vi "Get Cursor Values from Data.vi"(5 "spectra":cluster{"x0":dbl, "dx":dbl, "Y":dbl[]}[](array[cluster]), 7 "spectra info":T6[](array[typedef]) {"x-axis units" items=["Time (s)"=0, "Frequency-CB (Hz)"=1, "Frequency-CPB (Hz)"=1248, "Frequency-Arbitrary (Hz)"=2357, "Quefrency (s)"=2, "Revolutions (rev)"=3, "Order"=4, "Speed (RPM)"=11, "Speed (rad/s)"=21, "Index"=65535]; "weighting filter" items=["Linear", "A-weighting", "B-weighting", "C-weighting", "ITU-R 468-4", "Dolby", "CCITT", "C-message", "Wb", "Wc", "Wd", "We", "Wf", "Wh", "Wj", "Wk", "Wm", "AES17 20 kHz lowpass", "AES17 40 kHz lowpass", "AES17 20 kHz highpass", "AES17 40 kHz highpass"]; "dB reference [EU]" format="%.2f"; "engineering units" items=["custom..."=0, "V"=1, "A"=21, "C"=30, "pC"=31, "s"=32, "-"=29, "Pa"=2, "N"=20, "g"=3, "m/s^2"=4, "m/s"=5, "m"=6, "mm/s"=12, "mm"=13, "micron/s"=14, "micron"=15, "in/s^2"=7, "in/s"=8, "in"=9, "mil/s"=10, "mil"=11, "rad/s^2"=16, "rad/s"=17, "rad"=18, "deg/s^2"=26, "deg/s"=27, "deg"=28, "RPM"=22, "cycle/s^2"=23, "Hz"=24, "cycle"=25, "strain"=19]; "spectral info"."window" items=["None "=0, "Hanning"=1, "Hamming"=2, "Blackman-Harris"=3, "Exact Blackman"=4, "Blackman"=5, "Flat Top"=6, "4 Term B-Harris "=7, "7 Term B-Harris"=8, "Low Sidelobe"=9, "Force - Exponential"=10, "Gaussian"=62]}, 10 "Refnums for FP Objects":T1, 11 "Display State In":T2={"Graph Visible Items"={"Plot Legend"=FALSE, "Scale Legend"=FALSE, "Graph Palette"=FALSE, "Cursor Legend"=FALSE, "X Scrollbar"=FALSE}, "View Table"=FALSE, "Table Visible Items"={"Vertical Scrollbar"=FALSE, "Horizontal Scrollbar"=FALSE, "Row Headers"=FALSE, "Column Headers"=FALSE, "Vertical Lines"=FALSE, "Horizontal Lines"=FALSE}, "Header Font"={"Font Name"="", "Size"=0, "Bold"=FALSE, "Italic"=FALSE, "Underline"=FALSE, "Strikeout"=FALSE, "Color"=0}, "Cell Font"={"Font Name"="", "Size"=0, "Bold"=FALSE, "Italic"=FALSE, "Underline"=FALSE, "Strikeout"=FALSE, "Color"=0}, "Description and Tip..."={"Description"="", "Tip"=""}, "Moveable Splitter Position"=0, "Measurement Cursor Configuration"={"XY"={"enable XY"=FALSE, "Position (X)"=[], "Type"=enum."Absolute", "Y reference"=0.0, "color"=0}, "band"={"enable band"=FALSE, "B1"=0.0, "B2"=0.0, "Fixed bandwidth (B2-B1)"=0.0, "B1 color"=0, "B2 color"=0}, "harmonic"={"enable harmonics"=FALSE, "X reference (1X)"=0.0, "Maximum"=0, "Subset"=enum."All", "1X color"=0, "MX color"=0}, "sideband"={"enable sideband"=FALSE, "X center (C)"=0.0, "Sidebands"=0, "X spacing (s)"=0.0, "Center color"=0, "Sideband color"=0}}, "Cursors"={"List"=[], "Tags"=[]}, "X Increment"=0.0, "X Scale"={"Label Visible"=FALSE, "Label Text"="", "Mapping Mode"=0, "Format String"=""}, "Y Scale"={"Label Visible"=FALSE, "Label Text"="", "Mapping Mode"=0, "Format String"=""}, "Colors"={"background"=16777215, "major grid"=8355711, "minor grid"=12632256, "font"=0}, "desired spectrum view"={"scaling"={"linear/dB"=enum."no change", "dB reference"=0.0, "power/magnitude"=enum."no change", "view"=enum."no change"}, "spectral density"=enum."no change"}, "Plot Color Wheel"=[3381759, 32768, 982784, 4375295, 13827953, 13457919, 16757522, 4343295, 16728758, 12095254], "Plots"=[], "registered user events"=variant, "Lock 1X to Peak"=FALSE, "spectrum component"=32, "phase spectrum view"={"desired units"=0, "desired wrapping"=4}} caption="State" {"phase spectrum view"."desired wrapping" items=["No change", "Unwrap", "Wrap: -360 to 0", "Wrap: -270 to 90", "Wrap: -180 to 180", "Wrap: -90 to 270", "Wrap: 0 to 360", "Wrap: custom range"]; "phase spectrum view"."desired units" items=["No change", "Radians", "Degrees", "Cycles"]; "spectrum component" items=["Magnitude^2"=37, "Magnitude"=32, "Phase"=33, "Real"=34, "Imaginary"=35, "Coherence"=36, "Unknown"=99]; "Y Scale"."Mapping Mode" items=["Linear", "Logarithmic", "dB"]; "X Scale"."Mapping Mode" items=["Linear", "Logarithmic"]}) -> (2 "value table":string[][](array[string]), 3 "Display State Out":T2={"Graph Visible Items"={"Plot Legend"=FALSE, "Scale Legend"=FALSE, "Graph Palette"=FALSE, "Cursor Legend"=FALSE, "X Scrollbar"=FALSE}, "View Table"=FALSE, "Table Visible Items"={"Vertical Scrollbar"=FALSE, "Horizontal Scrollbar"=FALSE, "Row Headers"=FALSE, "Column Headers"=FALSE, "Vertical Lines"=FALSE, "Horizontal Lines"=FALSE}, "Header Font"={"Font Name"="", "Size"=0, "Bold"=FALSE, "Italic"=FALSE, "Underline"=FALSE, "Strikeout"=FALSE, "Color"=0}, "Cell Font"={"Font Name"="", "Size"=0, "Bold"=FALSE, "Italic"=FALSE, "Underline"=FALSE, "Strikeout"=FALSE, "Color"=0}, "Description and Tip..."={"Description"="", "Tip"=""}, "Moveable Splitter Position"=0, "Measurement Cursor Configuration"={"XY"={"enable XY"=FALSE, "Position (X)"=[], "Type"=enum."Absolute", "Y reference"=0.0, "color"=0}, "band"={"enable band"=FALSE, "B1"=0.0, "B2"=0.0, "Fixed bandwidth (B2-B1)"=0.0, "B1 color"=0, "B2 color"=0}, "harmonic"={"enable harmonics"=FALSE, "X reference (1X)"=0.0, "Maximum"=0, "Subset"=enum."All", "1X color"=0, "MX color"=0}, "sideband"={"enable sideband"=FALSE, "X center (C)"=0.0, "Sidebands"=0, "X spacing (s)"=0.0, "Center color"=0, "Sideband color"=0}}, "Cursors"={"List"=[], "Tags"=[]}, "X Increment"=0.0, "X Scale"={"Label Visible"=FALSE, "Label Text"="", "Mapping Mode"=0, "Format String"=""}, "Y Scale"={"Label Visible"=FALSE, "Label Text"="", "Mapping Mode"=0, "Format String"=""}, "Colors"={"background"=16777215, "major grid"=8355711, "minor grid"=12632256, "font"=0}, "desired spectrum view"={"scaling"={"linear/dB"=enum."no change", "dB reference"=0.0, "power/magnitude"=enum."no change", "view"=enum."no change"}, "spectral density"=enum."no change"}, "Plot Color Wheel"=[3381759, 32768, 982784, 4375295, 13827953, 13457919, 16757522, 4343295, 16728758, 12095254], "Plots"=[], "registered user events"=variant, "Lock 1X to Peak"=FALSE, "spectrum component"=32, "phase spectrum view"={"desired units"=0, "desired wrapping"=4}} caption="State" {"phase spectrum view"."desired wrapping" items=["No change", "Unwrap", "Wrap: -360 to 0", "Wrap: -270 to 90", "Wrap: -180 to 180", "Wrap: -90 to 270", "Wrap: 0 to 360", "Wrap: custom range"]; "phase spectrum view"."desired units" items=["No change", "Radians", "Degrees", "Cycles"]; "spectrum component" items=["Magnitude^2"=37, "Magnitude"=32, "Phase"=33, "Real"=34, "Imaginary"=35, "Coherence"=36, "Unknown"=99]; "Y Scale"."Mapping Mode" items=["Linear", "Logarithmic", "dB"]; "X Scale"."Mapping Mode" items=["Linear", "Logarithmic"]}, 4 "measurement names":string[](array[string]), 6 "channels":string[](array[string]))   [LabVIEW 2017, in "Spectrum with Cursors.xctl"]
doc: "This VI extracts the spectral values at the cursor positions. Based on the spectral data, Row Headers, Column Headers, and Values are written to the table."
uses:
  <vilib>/addons/_XControls/Spectrum with Cursors/Spectrum with Cursors.xctl
  <vilib>/addons/_XControls/Spectrum with Cursors/Controls/State.ctl
  <vilib>/Utility/miscctls.llb/LVFontTypeDef.ctl
  <vilib>/addons/_XControls/Spectrum with Cursors/Controls/Measurement Cursor Configuration.ctl
  <vilib>/addons/_NISVFA/_Shared subVIs/Controls/NI Spectrum Component.ctl
  <vilib>/addons/_NISVFA/_Shared subVIs/Controls/svc_Spectrum Info.ctl
  <vilib>/addons/_NISVFA/_Shared subVIs/Controls/svc_X-Axis Units.ctl
  <vilib>/addons/_NISVFA/_Shared subVIs/Controls/svc_Spectrum Type.ctl
  <vilib>/addons/_NISVFA/_Shared subVIs/Controls/svc_Engineering Units Text Ring.ctl
  <vilib>/addons/_NISVFA/_Shared subVIs/Controls/svc_Weighting Filter Text Ring.ctl
  <vilib>/addons/_NISVFA/_Shared subVIs/Controls/svc_Complimentary Spectrum Units.ctl
  <vilib>/addons/_XControls/Spectrum with Cursors/Controls/Refnums Typedef.ctl
  <vilib>/addons/_NISVFA/_Spectrum Processing/SVFA Get Spectrum Value (N Ch).vi
  <vilib>/Analysis/baseanly.llb/Mean (DBL).vi
  <vilib>/addons/_NISVFA/_Spectrum Processing/SVFA Get Spectrum Subset (N Ch).vi
  <vilib>/addons/_NISVFA/_Spectrum Processing/SVFA Power in Band (N Ch).vi
  <vilib>/addons/_NISVFA/_Spectrum Processing/SVFA Get Spectrum Value (1 Ch).vi
  <vilib>/addons/_NISVFA/_Spectrum Processing/SVFA Get Spectrum Subset (1 Ch).vi
  <vilib>/addons/_NISVFA/_Spectrum Processing/SVFA Power in Band (1 Ch).vi
  <vilib>/addons/_NISVFA/_Spectrum Processing/SVFA Unit Conversion.vi
  <vilib>/addons/_NISVFA/_Spectrum Processing/SVFA Unit Conversion (1 Ch).vi
  <vilib>/addons/_NISVFA/_Spectrum Processing/subVIs/svfa_Conversion Utility (spectrum info).vi
  <vilib>/addons/_NISVFA/_Spectrum Processing/subVIs/svfa_Peak to RMS to Peak2Peak.vi
  <vilib>/addons/_NISVFA/_Spectrum Processing/subVIs/svfa_Mag to Mag2.vi
  <vilib>/addons/_NISVFA/_Spectrum Processing/subVIs/svfa_Linear to dB.vi
  <vilib>/addons/_NISVFA/_Spectrum Processing/subVIs/svfa_dBrefA to dBrefB.vi
  <vilib>/addons/_NISVFA/_Spectrum Processing/subVIs/svfa_Spectrum to Spectral Density.vi
  <vilib>/addons/_NISVFA/_Shared subVIs/Common/svc_Caller VI Returned in Error Source.vi
  <vilib>/addons/_NISVFA/_Shared subVIs/Common/svc_Build Unit Label for Frequency Range.vi
  <vilib>/addons/_NISVFA/_Shared subVIs/Common/svc_Convert Frequency to Frequency String.vi
  <vilib>/addons/_NISVFA/_Shared subVIs/Common/svc_Check Frequency Range in Spectrum.vi
  <vilib>/addons/_NISVFA/_Shared subVIs/Common/svc_Get Weighting Enum and Labels.vi
  <vilib>/addons/_NISVFA/_Shared subVIs/Common/svc_Unit Label Lexical Class.vi
  <vilib>/addons/_NISVFA/_Shared subVIs/Common/svc_Engineering Units to Unit Label.vi
  <vilib>/addons/_NISVFA/_Shared subVIs/Common/svc_Format Value (DBL).vi
  <vilib>/Analysis/NI_AALBase.lvlib
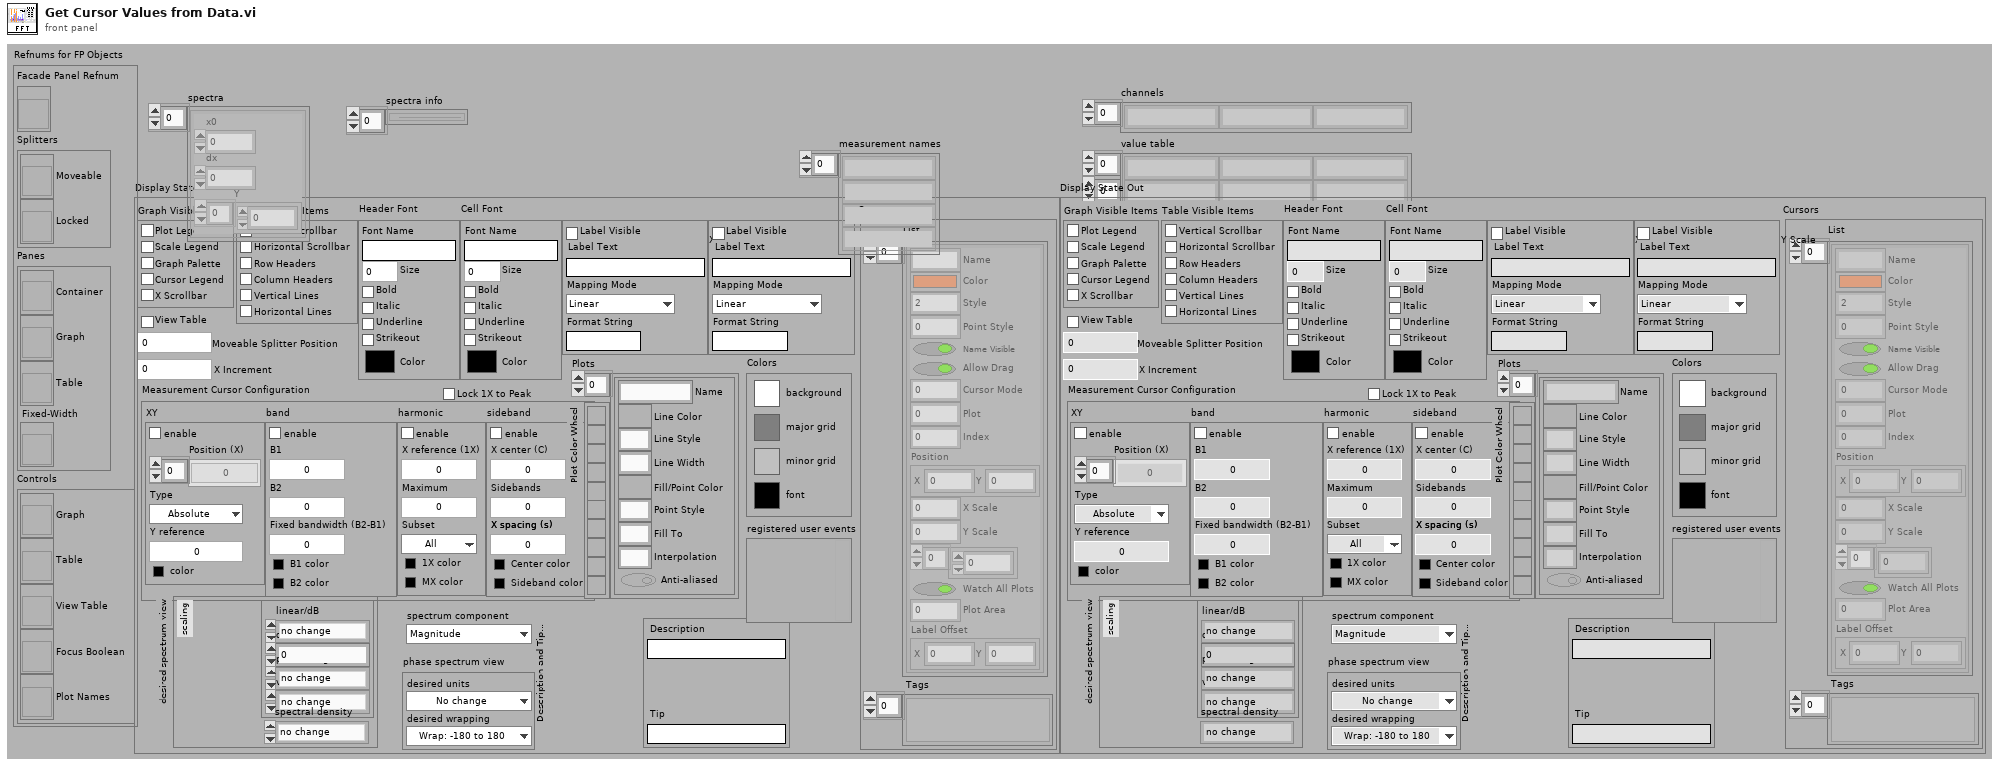
[diagram p1: front panel]
types:
  T1 = typedef "Spectrum with Cursors.xctl/Refnums Typedef.ctl" = cluster{"Facade Panel Refnum":refnum<vi>, "Splitters":cluster{"Moveable":refnum<vi>, "Locked":refnum<vi>}, "Panes":cluster{"Container":refnum<vi>, "Graph":refnum<vi>, "Table":refnum<vi>, "Fixed-Width":refnum<vi>}, "Controls":cluster{"Graph":refnum<vi>, "Table":refnum<vi>, "View Table":refnum<vi>, "Focus Boolean":refnum<vi>, "Plot Names":refnum<vi>}}
  T2 = typedef "Spectrum with Cursors.xctl/State.ctl" = cluster{"Graph Visible Items":cluster{"Plot Legend":bool, "Scale Legend":bool, "Graph Palette":bool, "Cursor Legend":bool, "X Scrollbar":bool}, "View Table":bool, "Table Visible Items":cluster{"Vertical Scrollbar":bool, "Horizontal Scrollbar":bool, "Row Headers":bool, "Column Headers":bool, "Vertical Lines":bool, "Horizontal Lines":bool}, "Header Font":T3, "Cell Font":T3, "Description and Tip...":cluster{"Description":string, "Tip":string}, "Moveable Splitter Position":i32, "Measurement Cursor Configuration":T4, "Cursors":cluster{"List":cluster{"Name":string, "Color":u32, "Style":i32, "Point Style":u8, "Name Visible":bool, "Allow Drag":bool, "Cursor Mode":u32, "Plot":i32, "Index":i32, "Position":cluster{"X":dbl, "Y":dbl}, "X Scale":u32, "Y Scale":u32, "Watch Plots":i32[], "Watch All Plots":bool, "Plot Area":i32, "Label Offset":cluster{"X":dbl, "Y":dbl}}[], "Tags":variant[]}, "X Increment":dbl, "X Scale":cluster{"Label Visible":bool, "Label Text":string, "Mapping Mode":u8, "Format String":string}, "Y Scale":cluster{"Label Visible":bool, "Label Text":string, "Mapping Mode":u8, "Format String":string}, "Colors":cluster{"background":u32, "major grid":u32, "minor grid":u32, "font":u32}, "desired spectrum view":cluster{"scaling":cluster{"linear/dB":enum16{"no change", "linear", "dB"}, "dB reference":dbl, "power/magnitude":enum16{"no change", "power", "magnitude"}, "view":enum16{"no change", "rms", "peak", "peak-peak"}}, "spectral density":enum16{"no change", "spectrum", "spectral density"}}, "Plot Color Wheel":u32[], "Plots":cluster{"Name":string, "Line Color":u32, "Line Style":u8, "Line Width":u8, "Fill/Point Color":u32, "Point Style":u8, "Fill To":i16, "Interpolation":u8, "Anti-aliased":bool}[], "registered user events":variant, "Lock 1X to Peak":bool, "spectrum component":T5, "phase spectrum view":cluster{"desired units":u16, "desired wrapping":u16}}
  T3 = typedef "LVFontTypeDef.ctl" = cluster{"Font Name":string, "Size":u16, "Bold":bool, "Italic":bool, "Underline":bool, "Strikeout":bool, "Color":u32}
  T4 = typedef "Spectrum with Cursors.xctl/Measurement Cursor Configuration.ctl" = cluster{"XY":cluster{"enable XY":bool, "Position (X)":dbl[], "Type":enum16{"Absolute", "Relative"}, "Y reference":dbl, "color":u32}, "band":cluster{"enable band":bool, "B1":dbl, "B2":dbl, "Fixed bandwidth (B2-B1)":dbl, "B1 color":u32, "B2 color":u32}, "harmonic":cluster{"enable harmonics":bool, "X reference (1X)":dbl, "Maximum":i32, "Subset":enum16{"All", "Even", "Odd"}, "1X color":u32, "MX color":u32}, "sideband":cluster{"enable sideband":bool, "X center (C)":dbl, "Sidebands":i32, "X spacing (s)":dbl, "Center color":u32, "Sideband color":u32}}
  T5 = typedef "NI Spectrum Component.ctl" = u16
  T6 = typedef "svc_Spectrum Info.ctl" = cluster{"channel name":string, "description":string, "x-axis units":T7, "spectral info":cluster{"spectrum type":T8, "linear/dB":enum16{"linear", "dB"}, "window":u16, "window size":i32, "FFT size":i32}, "engineering units":T9, "custom label":string, "dB reference [EU]":dbl, "peak units":enum16{"rms", "peak", "peak-peak"}, "weighting filter":T10, "spectral density?":bool, "unit label":string, "spectrum skewed?":bool, "complimentary spectrum units":T11}
  T7 = typedef "svc_X-Axis Units.ctl" = u16
  T8 = typedef "svc_Spectrum Type.ctl" = enum16{"FFT Spectrum [complex]", "Amplitude [Magnitude]", "Power [Magnitude^2]", "Cross Spectrum [complex]", "Frequency Response [Complex]"}
  T9 = typedef "svc_Engineering Units Text Ring.ctl" = u16
  T10 = typedef "svc_Weighting Filter Text Ring.ctl" = u16
  T11 = typedef "svc_Complimentary Spectrum Units.ctl" = enum16{"none", "radians", "degrees", "cycles", "imaginary"}
  T12 = enum16{"coerce to nearest", "coerce to next highest", "coerce to next lowest", "interpolate"}
  T13 = typedef "NI_AALPro.lvlib/windowTd.ctl" = u32
  T14 = cluster{"List":cluster{"Name":string, "Color":u32, "Style":i32, "Point Style":u8, "Name Visible":bool, "Allow Drag":bool, "Cursor Mode":u32, "Plot":i32, "Index":i32, "Position":cluster{"X":dbl, "Y":dbl}, "X Scale":u32, "Y Scale":u32, "Watch Plots":i32[], "Watch All Plots":bool, "Plot Area":i32, "Label Offset":cluster{"X":dbl, "Y":dbl}}[], "Tags":variant[]}
  T15 = cluster{"Name":string, "Color":u32, "Style":i32, "Point Style":u8, "Name Visible":bool, "Allow Drag":bool, "Cursor Mode":u32, "Plot":i32, "Index":i32, "Position":cluster{"X":dbl, "Y":dbl}, "X Scale":u32, "Y Scale":u32, "Watch Plots":i32[], "Watch All Plots":bool, "Plot Area":i32, "Label Offset":cluster{"X":dbl, "Y":dbl}}[]
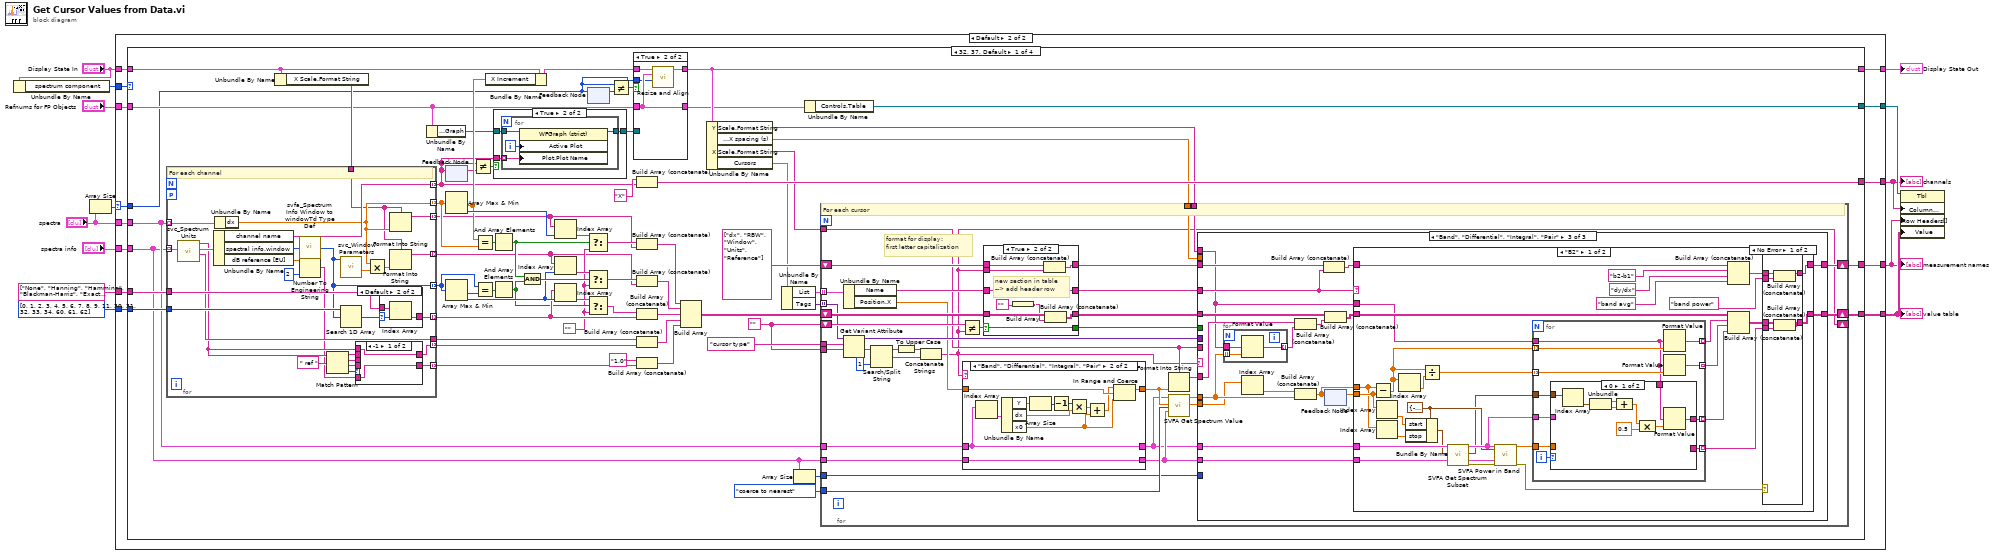
[diagram p0: block diagram]
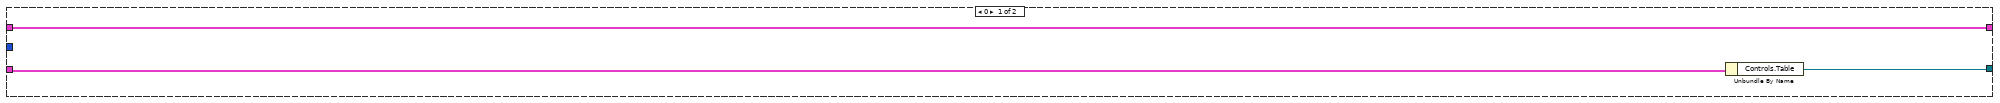
[diagram p2: hidden frame]
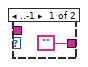
[diagram p6: hidden frame]
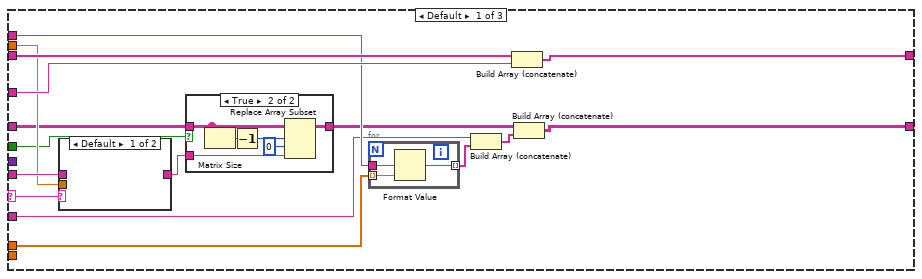
[diagram p9: hidden frame]
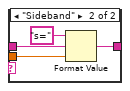
[diagram p11: hidden frame]
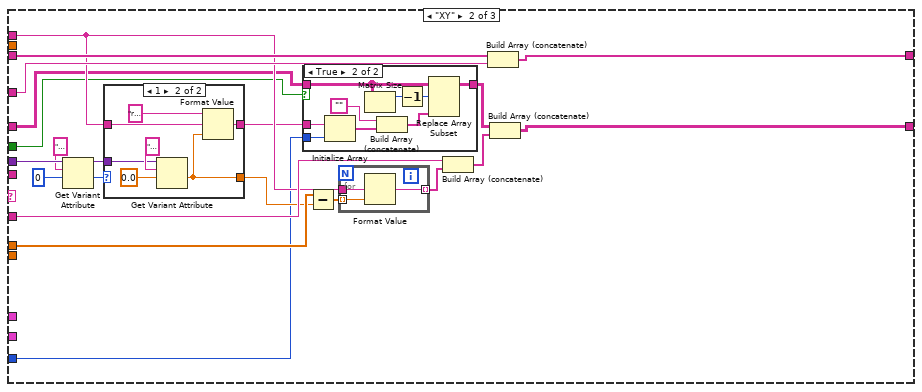
[diagram p12: hidden frame]
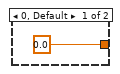
[diagram p14: hidden frame]
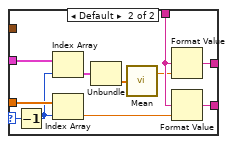
[diagram p16: hidden frame]
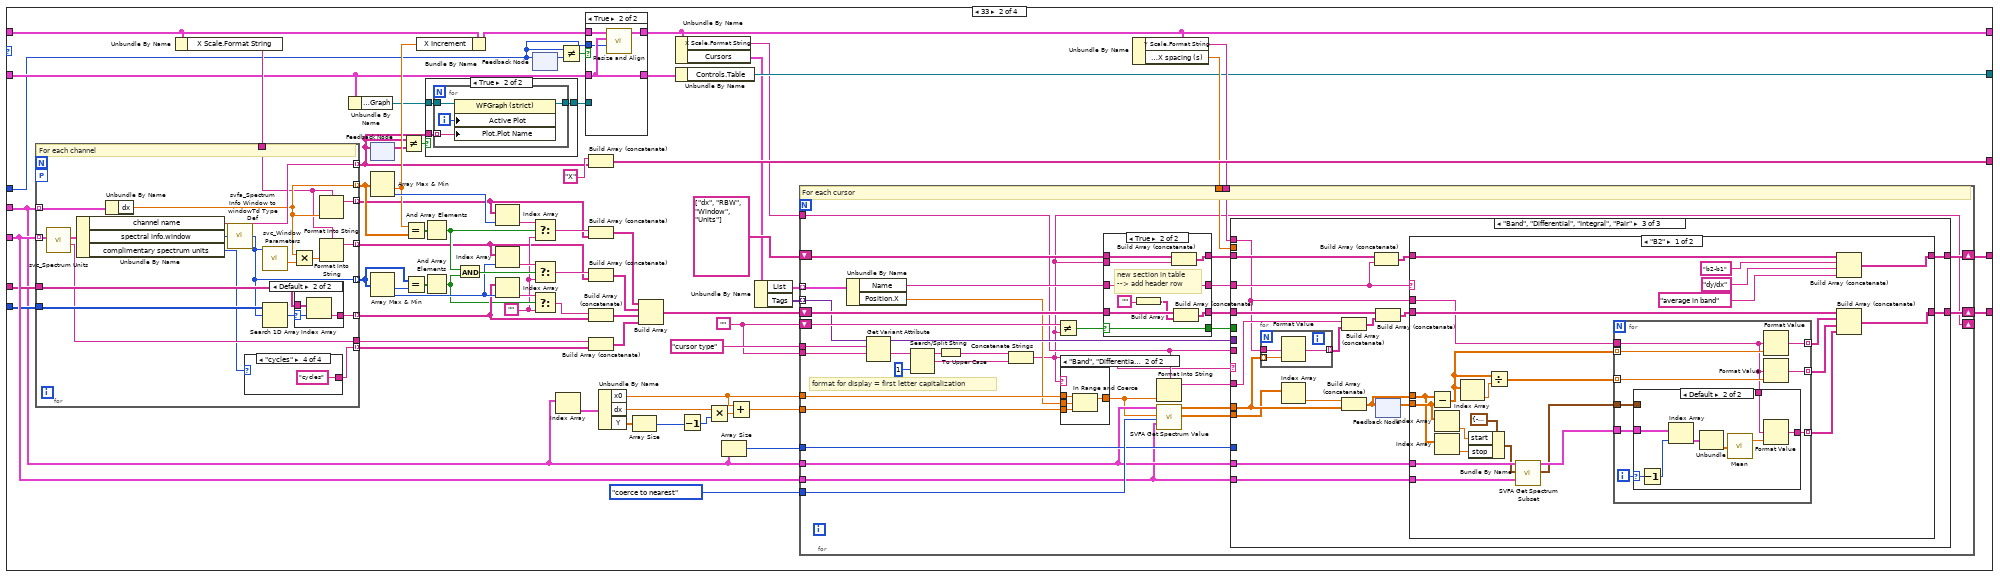
[diagram p18: hidden frame]
diagram:
  n1 = Unbundle By Name("Display State In") -> ("spectrum component"=w2:T5)
  n2 = Array Size(array="spectra") -> (size(s)=w7:i32)
  n3 = case shown="Default" w7 {
    selector: w7 -> [_ w18]
    tunnel: "spectra info" -> [_ w29]
    tunnel: u32[] [0, 1, 2, 3, 4, 5, 6, 7, 8, 9, 11, 30, 31, 32, 33, 34, 60, 61, 62] ("Array") -> [_ w28]
    tunnel: string[] ["None", "Hanning", "Hamming", "Blackman-Harris", "Exact Blackman", "Blackman", "Flat Top", "4 Term B-Harris ", "7 Term B-Harris", "Low Sidelobe", "Blackman Nuttall", "Triangle", "Bartlett-Hanning", "Bohman", "Parzen", "Welch", "Kaiser", "Dolph-Chebyshev", "Gaussian"] ("Array") -> [_ w27]
    tunnel: [_ w26] -> w4
    tunnel: [_ w25] -> w3
    tunnel: [_ w24] -> w5
    tunnel: [w16 w20] -> w10
    tunnel: "spectra" -> [_ w23]
    tunnel: "Display State In" -> [w16 w21]
    tunnel: "Refnums for FP Objects" -> [w15 w19]
    tunnel: [w14 w22] -> w6
    tunnel: w2 -> [_ w17]
    frame 0 {
      n4 = Unbundle By Name(w15) -> ("Controls.Table"=w14:refnum<vi>)
    }
    frame Default {
      n5 = case shown="32, 37, Default" w17 {
        tunnel: w29 -> [w32 w443 w753 w1061]
        tunnel: w28 -> [w93 w442 w752 w1060]
        tunnel: w27 -> [w92 w441 w751 w1059]
        tunnel: [w82 w431 w741 w1049] -> w26
        tunnel: [w81 w430 w740 w1048] -> w25
        tunnel: [w80 w429 w739 w1047] -> w24
        tunnel: w23 -> [w74 w415 w725 w1031]
        tunnel: [w51 w393 w703 w1008] -> w22
        tunnel: w21 -> [w48 w390 w700 w1005]
        tunnel: [w46 w388 w698 w1003] -> w20
        tunnel: w19 -> [w45 w387 w697 w1002]
        tunnel: w18 -> [w41 w383 w693 w998]
        frame 32, 37, Default {
          w79 = "" ("String")
          w56 = "" ("String")
          n6 = Unbundle By Name(w48) -> ("X Scale.Format String"=w50:string)
          n7 = for {
            tunnel: w32 -> [w135] mode=indexing
            tunnel: [w112] -> w33 mode=indexing
            tunnel: w74 -> [w136] mode=indexing
            tunnel: [w116] -> w89 mode=indexing
            tunnel: w93 -> [w132]
            tunnel: w92 -> [w129]
            tunnel: [w128] -> w36 mode=indexing
            tunnel: [w126] -> w37 mode=indexing
            tunnel: [w125] -> w60 mode=indexing
            tunnel: [w124] -> w90
            tunnel: [w114] -> w77 mode=indexing
            tunnel: w50 -> [w110]
            tunnel: [w111] -> w66 mode=indexing
            tunnel: [w109] -> w53 mode=indexing
            workers-P: _ -> [_]
            # "For each channel"
            n8 = call <vilib>:"svc_Spectrum Units.vi"("spectrum info in"=w135) -> ("x-axis unit label"=w124:string, "spectrum info out"=w134:T6, "unit label"=w115:string)  [unwired: 3 in, 1 out]
            n9 = Unbundle By Name(w134) -> ("channel name"=w112:string, "spectral info.window"=w131:u16, "dB reference [EU]"=w122:dbl)
            n10 = Unbundle By Name(w136) -> ("dx"=w111:dbl)
            n11 = call <vilib>:"svfa_Spectrum Info Window to windowTd Type Def.vi"("window"=w131) -> ("window"=w109:T13)  [unwired: 4 in]
            n12 = Number To Engineering String(2:i16 2 ("precision (6)"), 4:w122) -> (0:w113:string)  [unwired: 2 in]
            n13 = Match Pattern(string=w115, regular expression=" ref ") -> (before substring=w119:string, match substring=w118:string, after substring=w117:string, offset past match=w120:i32)  [unwired: 1 in]
            n14 = call <vilib>:"svc_Window Parameters.vi"("window"=w109) -> ("6dB BW"=w133:dbl)  [unwired: 7 in, 3 out]
            n15 = Search 1D Array(1D array=w132, element=w109) -> (index of element=w130:i32)  [unwired: 1 in]
            n16 = case shown="-1" w120 {
              tunnel: w119 -> [_ w140]
              tunnel: w118 -> [_ _]
              tunnel: w117 -> [_ w139]
              tunnel: [w138 w140] -> w116
              tunnel: w115 -> [w138 _]
              tunnel: [w137 w139] -> w114
              tunnel: w113 -> [w137 _]
              frame -1 {
              }
              frame Default {
              }
            }
            n17 = Multiply(x=w111, y=w133) -> (x*y=w127:dbl)
            n18 = case shown="Default" w130 {
              selector: w130 -> [_ w144]
              tunnel: w129 -> [_ w143]
              tunnel: ["" ("String") w142] -> w125
              frame ..-1 {
              }
              frame Default {
                n19 = Index Array(array=w143, index=w144) -> (element=w142:string)
              }
            }
            n20 = Format Into String(format string=w110, w111) -> (resulting string=w128:string)  [unwired: 2 in, 1 out]
            n21 = Format Into String(format string=w110, w127) -> (resulting string=w126:string)  [unwired: 2 in, 1 out]
          }
          n22 = Unbundle By Name(w45) -> ("Controls.Graph"=w52:refnum<vi>)
          n23 = feedback #1() -> (w35:string[])  [unwired: 1 in]
          n24 = feedback-in #1(w33) -> ()
          n25 = Array Max & Min(array=w66) -> (min value=w67:dbl, min index (indices)=w72:i32)  [unwired: 2 out]
          n26 = Array Max & Min(array=w53) -> (min value=w70:T13, min index (indices)=w63:i32)  [unwired: 2 out]
          n27 = Not Equal?(x=w33, y=w35) -> (x != y?=w34:bool)
          n28 = Equal?(x=w67, y=w66) -> (x = y?=w68:bool[])
          n29 = Equal?(x=w53, y=w70) -> (x = y?=w69:bool[])
          n30 = Bundle By Name(cluster=w48, "X Increment"=w67) -> (w47:T2)
          n31 = And Array Elements(Boolean array=w68) -> (logical AND=w57:bool)
          n32 = And Array Elements(Boolean array=w69) -> (logical AND=w59:bool)
          n33 = case shown="True" w34 {
            tunnel: w52 -> [w95 w98]
            tunnel: [w95 w97] -> w42
            tunnel: w33 -> [_ w96]
            frame False {
            }
            frame True {
              n34 = for {
                tunnel: w98 -> [w102]
                tunnel: w96 -> [w100] mode=indexing
                tunnel: [w99] -> w97
                i -> [w101]
                n35 = property class="WFGraph (strict)"(reference=w102, "Active Plot"=w101, "Plot.Plot Name"=w100) -> (reference out=w99:refnum<vi>)  [unwired: 1 in, 1 out]
              }
            }
          }
          n36 = And(x=w57, y=w59) -> (x .and. y?=w64:bool)
          n37 = Index Array(array=w36, index=w72) -> (element=w55:string)
          n38 = Index Array(array=w37, index=w63) -> (element=w65:string)
          n39 = Index Array(array=w60, index=w63) -> (element=w61:string)
          n40 = feedback #2() -> (w73:i32)  [unwired: 1 in]
          n41 = feedback-in #2(w41) -> ()
          n42 = Select(t=w55, s=w57, f=w56) -> (s? t:f=w54:string)
          n43 = Select(t=w65, s=w64, f=w56) -> (s? t:f=w62:string)
          n44 = Select(t=w61, s=w59, f=w56) -> (s? t:f=w58:string)
          n45 = Not Equal?(x=w41, y=w73) -> (x != y?=w43:bool)
          n46 = case shown="True" w43 {
            tunnel: w47 -> [w104 w108]
            tunnel: [w104 w107] -> w46
            tunnel: w45 -> [w103 w106]
            tunnel: [w103 w106] -> w44
            tunnel: w41 -> [_ w105]
            tunnel: w42 -> [_ _]
            frame False {
            }
            frame True {
              n47 = call <vilib>:"Resize and Align.vi"("number of channels"=w105, "Refnums for Resizing and Alignment"=w106, "State in"=w108) -> ("State out"=w107:T2)  [unwired: 7 in, 1 out]
            }
          }
          n48 = Build Array (concatenate)("X" ("String"), w33) -> (w80:string[])
          n49 = Build Array (concatenate)(w54, w36) -> (w84:string[])
          n50 = Build Array (concatenate)(w62, w37) -> (w87:string[])
          n51 = Build Array (concatenate)(w58, w60) -> (w83:string[])
          n52 = Build Array (concatenate)(w90, w89) -> (w88:string[])
          n53 = Build Array (concatenate)("1.0" ("String"), w77) -> (w78:string[])
          n54 = Build Array(w84, w87, w83, w88, w78) -> (w76:string[][])
          n55 = Unbundle By Name(w46) -> ("Y Scale.Format String"=w31:string, "Measurement Cursor Configuration.sideband.X spacing (s)"=w30:dbl, "X Scale.Format String"=w49:string, "Cursors"=w40:T14)
          n56 = Unbundle By Name(w40) -> ("List"=w39:T15, "Tags"=w38:variant[])
          n57 = Array Size(array=w32) -> (size(s)=w75:i32)
          n58 = Unbundle By Name(w44) -> ("Controls.Table"=w51:refnum<vi>)
          n59 = for {
            tunnel: w74 -> [w145]
            tunnel: w32 -> [w147]
            tunnel: T12."coerce to nearest" ("frequency coercion") -> [w180]
            shift-right: [w178] -> w81
            shift-left: string[] ["dx", "RBW", "Window", "Units", "Reference"] ("Array") -> [w170]
            shift-right: [w177] -> w82
            shift-left: w76 -> [w171]
            tunnel: "cursor type" -> [w176]
            shift-right: [w149] -> _
            shift-left: w79 -> [w175]
            tunnel: w79 -> [w174]
            tunnel: w49 -> [w150]
            tunnel: w31 -> [w160]
            tunnel: w75 -> [w158]
            tunnel: w30 -> [w157]
            tunnel: w39 -> [w154] mode=indexing
            tunnel: w38 -> [w151] mode=indexing
            # "format for display:\nfirst letter capitalization"
            # "For each cursor"
            n60 = Get Variant Attribute(Variant=w151, name=w176, default value (empty Variant)=w174) -> (duplicate Variant=w162:variant, value=w163:string)  [unwired: 1 in, 2 out]
            n61 = Unbundle By Name(w154) -> ("Name"=w153:string, "Position.X"=w152:dbl)
            n62 = Search/Split String(string=w163, offset (0)=1) -> (substring before match=w166:string, match + rest of string=w164:string)  [unwired: 1 in, 1 out]
            n63 = To Upper Case(1:w166) -> (0:w165:string)
            n64 = Concatenate Strings(w165, w164) -> (w149:string)
            n65 = Not Equal?(x=w175, y=w149) -> (x != y?=w173:bool)
            n66 = case shown="\"Band\", \"Differential\", \"Integral\", \"Pair\"" w149 {
              tunnel: w152 -> [w183 w195]
              tunnel: [w183 w194] -> w155
              tunnel: [w181 w193] -> w148
              tunnel: w147 -> [w181 w193]
              tunnel: [w182 w187] -> w146
              tunnel: w145 -> [w182 w187]
              frame Default {
              }
              frame "Band", "Differential", "Integral", "Pair" {
                n67 = Index Array(array=w187) -> (element=w188:cluster{"x0":dbl, "dx":dbl, "Y":dbl[]})  [unwired: 1 in]
                n68 = Unbundle By Name(w188) -> ("Y"=w189:dbl[], "dx"=w185:dbl, "x0"=w184:dbl)
                n69 = Array Size(array=w189) -> (size(s)=w190:i32)
                n70 = Decrement(x=w190) -> (x-1=w191:i32)
                n71 = Multiply(x=w191, y=w185) -> (x*y=w192:dbl)
                n72 = Add(x=w192, y=w184) -> (x+y=w186:dbl)
                n73 = In Range and Coerce(upper limit=w186, x=w195, lower limit=w184) -> (coerced(x)=w194:dbl)  [unwired: 1 out]
              }
            }
            n74 = case shown="True" w173 {
              selector: w173 -> [w196 w200]
              tunnel: [w199 w208] -> w172
              tunnel: w153 -> [w199 w208]
              tunnel: w171 -> [w197 w203]
              tunnel: w170 -> [w198 w206]
              tunnel: [w198 w207] -> w169
              tunnel: [w197 w204] -> w168
              tunnel: w149 -> [_ w205]
              tunnel: [w196 w200] -> w159
              frame False {
              }
              frame True {
                # "new section in table\n--> add header row"
                n75 = Build Array("") -> (w201:string[])
                n76 = Build Array (concatenate)(w206, w205) -> (w207:string[])
                n77 = Build Array (concatenate)(w203, w201) -> (w204:string[][])
              }
            }
            n78 = Format Into String(format string=w150, w155) -> (resulting string=w161:string)  [unwired: 2 in, 1 out]
            n79 = call-poly <vilib>:"SVFA Get Spectrum Value.vi"("spectra"=w146, "x value (1000)"=w155, "coercion (nearest)"=w180, "spectrum info"=w148) -> ("spectra values"=w179:dbl[], "actual x values"=w156:dbl[])  [unwired: 11 in, 3 out]
            n80 = case shown="\"Band\", \"Differential\", \"Integral\", \"Pair\"" w149 {
              selector: w149 -> [w216 _ _]
              tunnel: w179 -> [w218 w255 w293]
              tunnel: w169 -> [w224 w259 w298]
              tunnel: w172 -> [w223 w258 w292]
              tunnel: [w222 w257 w291] -> w178
              tunnel: w168 -> [w212 w242 w297]
              tunnel: [w221 w256 w288] -> w177
              tunnel: w162 -> [_ w254 _]
              tunnel: w161 -> [w215 w249 w295]
              tunnel: w160 -> [w219 w244 w283]
              tunnel: w159 -> [w210 w243 _]
              tunnel: w158 -> [_ w239 _]
              tunnel: w150 -> [w214 _ _]
              tunnel: w157 -> [w213 _ _]
              tunnel: w156 -> [_ _ w287]
              tunnel: w146 -> [_ _ w282]
              tunnel: w148 -> [_ _ w281]
              frame Default {
                n81 = case shown="Default" w216 {
                  tunnel: w214 -> [_ w234]
                  tunnel: w213 -> [_ w233]
                  tunnel: [_ w232] -> w209
                  frame Default {
                  }
                  frame "Sideband" {
                    n82 = Format Value(string ("")="s=", format string=w234, value (0)=w233) -> (output string=w232:string)
                  }
                }
                n83 = case shown="True" w210 {
                  tunnel: w212 -> [w225 w229]
                  tunnel: [w225 w231] -> w211
                  tunnel: w209 -> [_ w227]
                  frame False {
                  }
                  frame True {
                    n84 = Matrix Size(0:w229) -> (1:w230:i32)  [unwired: 1 out]
                    n85 = Decrement(x=w230) -> (x-1=w228:i32)
                    n86 = Replace Array Subset(array=w229, new element=w227, index (row)=w228, index (col)=0 ("disabled index (col)")) -> (w231:string[][])
                  }
                }
                n87 = for {
                  tunnel: w218 -> [w238] mode=indexing
                  tunnel: [w237] -> w220 mode=indexing
                  tunnel: w219 -> [w236]
                  n88 = Format Value(format string=w236, value (0)=w238) -> (output string=w237:string)  [unwired: 1 in]
                }
                n89 = Build Array (concatenate)(w215, w220) -> (w217:string[])
                n90 = Build Array (concatenate)(w224, w223) -> (w222:string[])
                n91 = Build Array (concatenate)(w211, w217) -> (w221:string[][])
              }
              frame "XY" {
                n92 = Get Variant Attribute(Variant=w254, name="xy type", default value (empty Variant)=u16 0 ("precision (6)")) -> (duplicate Variant=w253:variant, value=w250:u16)  [unwired: 1 in, 2 out]
                n93 = case shown="1" w250 {
                  tunnel: [0.0 ("element") w275] -> w247
                  tunnel: w253 -> [_ w278]
                  tunnel: w244 -> [_ w276]
                  tunnel: [_ w274] -> w240
                  frame 0, Default {
                  }
                  frame 1 {
                    n94 = Get Variant Attribute(Variant=w278, name="y reference", default value (empty Variant)=0.0 ("element")) -> (value=w275:dbl)  [unwired: 1 in, 3 out]
                    n95 = Format Value(string ("")="ref=", format string=w276, value (0)=w275) -> (output string=w274:string)
                  }
                }
                n96 = case shown="True" w243 {
                  tunnel: w242 -> [w260 w265]
                  tunnel: [w260 w269] -> w241
                  tunnel: w240 -> [_ w268]
                  tunnel: w239 -> [_ w267]
                  frame False {
                  }
                  frame True {
                    n97 = Initialize Array(w268, w267) -> (w263:string[])
                    n98 = Matrix Size(0:w265) -> (1:w266:i32)  [unwired: 1 out]
                    n99 = Build Array (concatenate)("", w263) -> (w261:string[])
                    n100 = Decrement(x=w266) -> (x-1=w264:i32)
                    n101 = Replace Array Subset(array=w265, new element=w261, index (row)=w264) -> (w269:string[][])  [unwired: 1 in]
                  }
                }
                n102 = Subtract(x=w255, y=w247) -> (x-y=w246:dbl[])
                n103 = for {
                  tunnel: w246 -> [w272] mode=indexing
                  tunnel: [w271] -> w245 mode=indexing
                  tunnel: w244 -> [w270]
                  n104 = Format Value(format string=w270, value (0)=w272) -> (output string=w271:string)  [unwired: 1 in]
                }
                n105 = Build Array (concatenate)(w249, w245) -> (w248:string[])
                n106 = Build Array (concatenate)(w259, w258) -> (w257:string[])
                n107 = Build Array (concatenate)(w241, w248) -> (w256:string[][])
              }
              frame "Band", "Differential", "Integral", "Pair" {
                n108 = for {
                  tunnel: w293 -> [w374] mode=indexing
                  tunnel: [w373] -> w296 mode=indexing
                  tunnel: w283 -> [w372]
                  n109 = Format Value(format string=w372, value (0)=w374) -> (output string=w373:string)  [unwired: 1 in]
                }
                n110 = Index Array(array=w287) -> (element=w286:dbl)  [unwired: 1 in]
                n111 = Build Array (concatenate)(w295, w296) -> (w294:string[])
                n112 = Build Array (concatenate)(w286, w293) -> (w285:dbl[])
                n113 = Build Array (concatenate)(w298, w292) -> (w290:string[])
                n114 = Build Array (concatenate)(w297, w294) -> (w289:string[][])
                n115 = feedback-in #3(w285) -> ()
                n116 = feedback #3() -> (w284:dbl[])  [unwired: 1 in]
                n117 = case shown="\"B2\"" w292 {
                  tunnel: [w305 w371] -> w291
                  tunnel: w290 -> [w330 w371]
                  tunnel: w289 -> [w328 w370]
                  tunnel: [w302 w370] -> w288
                  tunnel: w285 -> [w314 _]
                  tunnel: w284 -> [w316 _]
                  tunnel: w283 -> [w326 _]
                  tunnel: w282 -> [w320 _]
                  tunnel: w281 -> [w319 _]
                  frame "B2" {
                    w309 = cluster{"start":dbl, "stop":dbl} {"start"=-1.0, "stop"=-1.0} ("range")
                    n118 = Subtract(x=w314, y=w316) -> (x-y=w324:dbl[])
                    n119 = Index Array(array=w316) -> (element=w315:dbl)  [unwired: 1 in]
                    n120 = Index Array(array=w314) -> (element=w313:dbl)  [unwired: 1 in]
                    n121 = Index Array(array=w324) -> (element=w325:dbl)  [unwired: 1 in]
                    n122 = Bundle By Name(cluster=w309, "start"=w315, "stop"=w313) -> (w317:cluster{"start":dbl, "stop":dbl})
                    n123 = Divide(x=w324, y=w325) -> (x/y=w323:dbl[])
                    n124 = call-poly <vilib>:"SVFA Get Spectrum Subset.vi"("spectra"=w320, "range"=w317, "spectrum info"=w319) -> ("spectra subsets"=w312:cluster{"x0":dbl, "dx":dbl, "magnitude":dbl[]}[], "actual ranges"=w308:cluster{"start":dbl, "stop":dbl}[], "dup spectrum info"=w318:T6[], "error out"=w299:errorcluster)  [unwired: 11 in, 2 out]
                    n125 = call-poly <vilib>:"SVFA Power in Band.vi"("spectra"=w312, "range"=w309, "spectrum info"=w318, "error in (no error)"=w299) -> ("powers in band"=w311:dbl[], "error out"=w300:errorcluster)  [unwired: 13 in, 1 out]
                    n126 = for {
                      tunnel: w324 -> [w349] mode=indexing
                      tunnel: [w348] -> w327 mode=indexing
                      tunnel: w326 -> [w342]
                      tunnel: w323 -> [w347] mode=indexing
                      tunnel: [w346] -> w322 mode=indexing
                      tunnel: w312 -> [w344]
                      tunnel: w311 -> [w343]
                      tunnel: [w341] -> w301 mode=indexing
                      tunnel: [w340] -> w310 mode=indexing
                      tunnel: w308 -> [w339]
                      i -> [w345]
                      n127 = case shown="0" w345 {
                        selector: w345 -> [_ w369]
                        tunnel: w344 -> [_ w368]
                        tunnel: w343 -> [_ w367]
                        tunnel: w342 -> [w352 w366]
                        tunnel: [_ w364] -> w341
                        tunnel: [w351 w363] -> w340
                        tunnel: w339 -> [w358 _]
                        frame 0 {
                          n128 = Index Array(array=w358) -> (element=w350:cluster{"start":dbl, "stop":dbl})  [unwired: 1 in]
                          n129 = Unbundle(w350) -> ("start"=w357:dbl, "stop"=w356:dbl)
                          n130 = Compound Arithmetic op=ADD(w357, w356) -> (w355:dbl)
                          n131 = Compound Arithmetic op=MULTIPLY(w355, 0.5 ("value")) -> (w353:dbl)
                          n132 = Format Value(format string=w352, value (0)=w353) -> (output string=w351:string)  [unwired: 1 in]
                        }
                        frame Default {
                          n133 = Decrement(x=w369) -> (x-1=w359:i32)
                          n134 = Index Array(array=w368, index=w359) -> (element=w362:cluster{"x0":dbl, "dx":dbl, "magnitude":dbl[]})
                          n135 = Index Array(array=w367, index=w359) -> (element=w365:dbl)
                          n136 = Unbundle(w362) -> ("magnitude"=w361:dbl[])  [unwired: 2 out]
                          n137 = call-poly <vilib>:"Mean.vi"("X"=w361) -> ("mean"=w360:dbl)  [unwired: 1 out]
                          n138 = Format Value(format string=w366, value (0)=w360) -> (output string=w363:string)  [unwired: 1 in]
                          n139 = Format Value(format string=w366, value (0)=w365) -> (output string=w364:string)  [unwired: 1 in]
                        }
                      }
                      n140 = Format Value(format string=w342, value (0)=w349) -> (output string=w348:string)  [unwired: 1 in]
                      n141 = Format Value(format string=w342, value (0)=w347) -> (output string=w346:string)  [unwired: 1 in]
                    }
                    n142 = Build Array (concatenate)(w330, "b2-b1", "dy/dx", "band avg") -> (w306:string[])
                    n143 = Build Array (concatenate)(w328, w327, w322, w310) -> (w303:string[][])
                    n144 = case shown="No Error" w300 {
                      tunnel: w306 -> [w336 w338]
                      tunnel: [w335 w338] -> w305
                      tunnel: "band power" -> [w334 _]
                      tunnel: w303 -> [w333 w337]
                      tunnel: [w332 w337] -> w302
                      tunnel: w301 -> [w331 _]
                      frame No Error {
                        n145 = Build Array (concatenate)(w336, w334) -> (w335:string[])
                        n146 = Build Array (concatenate)(w333, w331) -> (w332:string[][])
                      }
                      frame Error {
                      }
                    }
                  }
                  frame "B1", Default {
                  }
                }
              }
            }
          }
        }
        frame 33 {
          w428 = "" ("String")
          w398 = "" ("String")
          n147 = Unbundle By Name(w390) -> ("X Scale.Format String"=w392:string)
          n148 = for {
            tunnel: w443 -> [w476] mode=indexing
            tunnel: [w464] -> w375 mode=indexing
            tunnel: w415 -> [w477] mode=indexing
            tunnel: [w459] -> w438 mode=indexing
            tunnel: w442 -> [w473]
            tunnel: w441 -> [w470]
            tunnel: [w469] -> w378 mode=indexing
            tunnel: [w467] -> w379 mode=indexing
            tunnel: [w466] -> w402 mode=indexing
            tunnel: [w465] -> w439
            tunnel: w392 -> [w462]
            tunnel: [w463] -> w408 mode=indexing
            tunnel: [w461] -> w395 mode=indexing
            workers-P: _ -> [_]
            # "For each channel"
            n149 = call <vilib>:"svc_Spectrum Units.vi"("spectrum info in"=w476) -> ("x-axis unit label"=w465:string, "spectrum info out"=w475:T6)  [unwired: 3 in, 2 out]
            n150 = Unbundle By Name(w475) -> ("channel name"=w464:string, "spectral info.window"=w472:u16, "complimentary spectrum units"=w460:T11)
            n151 = Unbundle By Name(w477) -> ("dx"=w463:dbl)
            n152 = call <vilib>:"svfa_Spectrum Info Window to windowTd Type Def.vi"("window"=w472) -> ("window"=w461:T13)  [unwired: 4 in]
            n153 = case shown="\"cycles\"" w460 {
              tunnel: ["" ("String") "rad" ("String") "deg" ("String") "cycles" ("String")] -> w459
              frame Default {
              }
              frame "radians" {
              }
              frame "degrees" {
              }
              frame "cycles" {
              }
            }
            n154 = call <vilib>:"svc_Window Parameters.vi"("window"=w461) -> ("6dB BW"=w474:dbl)  [unwired: 7 in, 3 out]
            n155 = Search 1D Array(1D array=w473, element=w461) -> (index of element=w471:i32)  [unwired: 1 in]
            n156 = Multiply(x=w463, y=w474) -> (x*y=w468:dbl)
            n157 = case shown="Default" w471 {
              selector: w471 -> [_ w485]
              tunnel: w470 -> [_ w484]
              tunnel: ["" ("String") w483] -> w466
              frame ..-1 {
              }
              frame Default {
                n158 = Index Array(array=w484, index=w485) -> (element=w483:string)
              }
            }
            n159 = Format Into String(format string=w462, w463) -> (resulting string=w469:string)  [unwired: 2 in, 1 out]
            n160 = Format Into String(format string=w462, w468) -> (resulting string=w467:string)  [unwired: 2 in, 1 out]
          }
          n161 = Unbundle By Name(w387) -> ("Controls.Graph"=w394:refnum<vi>)
          n162 = feedback #4() -> (w377:string[])  [unwired: 1 in]
          n163 = feedback-in #4(w375) -> ()
          n164 = Array Max & Min(array=w408) -> (min value=w409:dbl, min index (indices)=w413:i32)  [unwired: 2 out]
          n165 = Array Max & Min(array=w395) -> (min value=w412:T13, min index (indices)=w405:i32)  [unwired: 2 out]
          n166 = Not Equal?(x=w375, y=w377) -> (x != y?=w376:bool)
          n167 = Equal?(x=w409, y=w408) -> (x = y?=w410:bool[])
          n168 = Equal?(x=w395, y=w412) -> (x = y?=w411:bool[])
          n169 = Bundle By Name(cluster=w390, "X Increment"=w409) -> (w389:T2)
          n170 = And Array Elements(Boolean array=w410) -> (logical AND=w399:bool)
          n171 = And Array Elements(Boolean array=w411) -> (logical AND=w401:bool)
          n172 = case shown="True" w376 {
            tunnel: w394 -> [w445 w448]
            tunnel: [w445 w447] -> w384
            tunnel: w375 -> [_ w446]
            frame False {
            }
            frame True {
              n173 = for {
                tunnel: w448 -> [w452]
                tunnel: w446 -> [w450] mode=indexing
                tunnel: [w449] -> w447
                i -> [w451]
                n174 = property class="WFGraph (strict)"(reference=w452, "Active Plot"=w451, "Plot.Plot Name"=w450) -> (reference out=w449:refnum<vi>)  [unwired: 1 in, 1 out]
              }
            }
          }
          n175 = And(x=w399, y=w401) -> (x .and. y?=w406:bool)
          n176 = Index Array(array=w378, index=w413) -> (element=w397:string)
          n177 = Index Array(array=w379, index=w405) -> (element=w407:string)
          n178 = Index Array(array=w402, index=w405) -> (element=w403:string)
          n179 = feedback #5() -> (w414:i32)  [unwired: 1 in]
          n180 = feedback-in #5(w383) -> ()
          n181 = Select(t=w397, s=w399, f=w398) -> (s? t:f=w396:string)
          n182 = Select(t=w407, s=w406, f=w398) -> (s? t:f=w404:string)
          n183 = Select(t=w403, s=w401, f=w398) -> (s? t:f=w400:string)
          n184 = Index Array(array=w415) -> (element=w423:cluster{"x0":dbl, "dx":dbl, "Y":dbl[]})  [unwired: 1 in]
          n185 = Not Equal?(x=w383, y=w414) -> (x != y?=w385:bool)
          n186 = case shown="True" w385 {
            tunnel: w389 -> [w454 w458]
            tunnel: [w454 w457] -> w388
            tunnel: w387 -> [w453 w456]
            tunnel: [w453 w456] -> w386
            tunnel: w383 -> [_ w455]
            tunnel: w384 -> [_ _]
            frame False {
            }
            frame True {
              n187 = call <vilib>:"Resize and Align.vi"("number of channels"=w455, "Refnums for Resizing and Alignment"=w456, "State in"=w458) -> ("State out"=w457:T2)  [unwired: 7 in, 1 out]
            }
          }
          n188 = Build Array (concatenate)("X" ("String"), w375) -> (w429:string[])
          n189 = Build Array (concatenate)(w396, w378) -> (w433:string[])
          n190 = Build Array (concatenate)(w404, w379) -> (w436:string[])
          n191 = Build Array (concatenate)(w400, w402) -> (w432:string[])
          n192 = Build Array (concatenate)(w439, w438) -> (w437:string[])
          n193 = Unbundle By Name(w423) -> ("x0"=w416:dbl, "dx"=w419:dbl, "Y"=w422:dbl[])
          n194 = Array Size(array=w422) -> (size(s)=w421:i32)
          n195 = Build Array(w433, w436, w432, w437) -> (w426:string[][])
          n196 = Unbundle By Name(w388) -> ("X Scale.Format String"=w391:string, "Cursors"=w382:T14)
          n197 = Unbundle By Name(w386) -> ("Controls.Table"=w393:refnum<vi>)
          n198 = Decrement(x=w421) -> (x-1=w420:i32)
          n199 = Multiply(x=w419, y=w420) -> (x*y=w418:dbl)
          n200 = Array Size(array=w415) -> (size(s)=w425:i32)
          n201 = Add(x=w416, y=w418) -> (x+y=w417:dbl)
          n202 = Unbundle By Name(w382) -> ("List"=w381:T15, "Tags"=w380:variant[])
          n203 = Unbundle By Name(w388) -> ("Y Scale.Format String"=w427:string, "Measurement Cursor Configuration.sideband.X spacing (s)"=w424:dbl)
          n204 = for {
            tunnel: w415 -> [w496]
            tunnel: w443 -> [w495]
            tunnel: T12."coerce to nearest" ("frequency coercion") -> [w521]
            shift-right: [w519] -> w430
            shift-left: string[] ["dx", "RBW", "Window", "Units"] ("Array") -> [w511]
            shift-right: [w518] -> w431
            shift-left: w426 -> [w512]
            tunnel: "cursor type" -> [w517]
            shift-right: [w486] -> _
            shift-left: w428 -> [w516]
            tunnel: w428 -> [w515]
            tunnel: w391 -> [w487]
            tunnel: w427 -> [w501]
            tunnel: w425 -> [w499]
            tunnel: w424 -> [w498]
            tunnel: w417 -> [w493]
            tunnel: w416 -> [w492]
            tunnel: w381 -> [w491] mode=indexing
            tunnel: w380 -> [w488] mode=indexing
            # "format for display = first letter capitalization"
            # "For each cursor"
            n205 = Unbundle By Name(w491) -> ("Name"=w490:string, "Position.X"=w489:dbl)
            n206 = Get Variant Attribute(Variant=w488, name=w517, default value (empty Variant)=w515) -> (duplicate Variant=w503:variant, value=w504:string)  [unwired: 1 in, 2 out]
            n207 = Search/Split String(string=w504, offset (0)=1) -> (substring before match=w507:string, match + rest of string=w505:string)  [unwired: 1 in, 1 out]
            n208 = To Upper Case(1:w507) -> (0:w506:string)
            n209 = Concatenate Strings(w506, w505) -> (w486:string)
            n210 = Not Equal?(x=w516, y=w486) -> (x != y?=w514:bool)
            n211 = case shown="\"Band\", \"Differential\", \"Integral\", \"Pair\"" w486 {
              tunnel: w489 -> [w522 w526]
              tunnel: [w522 w525] -> w494
              tunnel: w493 -> [_ w524]
              tunnel: w492 -> [_ w523]
              frame Default {
              }
              frame "Band", "Differential", "Integral", "Pair" {
                n212 = In Range and Coerce(upper limit=w523, x=w526, lower limit=w524) -> (coerced(x)=w525:dbl)  [unwired: 1 out]
              }
            }
            n213 = case shown="True" w514 {
              selector: w514 -> [w527 w531]
              tunnel: [w530 w539] -> w513
              tunnel: w490 -> [w530 w539]
              tunnel: w512 -> [w528 w534]
              tunnel: w511 -> [w529 w537]
              tunnel: [w529 w538] -> w510
              tunnel: [w528 w535] -> w509
              tunnel: w486 -> [_ w536]
              tunnel: [w527 w531] -> w500
              frame False {
              }
              frame True {
                # "new section in table\n--> add header row"
                n214 = Build Array("") -> (w532:string[])
                n215 = Build Array (concatenate)(w537, w536) -> (w538:string[])
                n216 = Build Array (concatenate)(w534, w532) -> (w535:string[][])
              }
            }
            n217 = Format Into String(format string=w487, w494) -> (resulting string=w502:string)  [unwired: 2 in, 1 out]
            n218 = call-poly <vilib>:"SVFA Get Spectrum Value.vi"("spectra"=w496, "x value (1000)"=w494, "coercion (nearest)"=w521, "spectrum info"=w495) -> ("spectra values"=w520:dbl[], "actual x values"=w497:dbl[])  [unwired: 11 in, 3 out]
            n219 = case shown="\"Band\", \"Differential\", \"Integral\", \"Pair\"" w486 {
              selector: w486 -> [w547 _ _]
              tunnel: w520 -> [w549 w586 w624]
              tunnel: w510 -> [w555 w590 w629]
              tunnel: w513 -> [w554 w589 w623]
              tunnel: [w553 w588 w622] -> w519
              tunnel: w509 -> [w543 w573 w628]
              tunnel: [w552 w587 w619] -> w518
              tunnel: w503 -> [_ w585 _]
              tunnel: w502 -> [w546 w580 w626]
              tunnel: w501 -> [w550 w575 w614]
              tunnel: w500 -> [w541 w574 _]
              tunnel: w499 -> [_ w570 _]
              tunnel: w487 -> [w545 _ _]
              tunnel: w498 -> [w544 _ _]
              tunnel: w497 -> [_ _ w618]
              tunnel: w496 -> [_ _ w613]
              tunnel: w495 -> [_ _ w612]
              frame Default {
                n220 = case shown="\"Sideband\"" w547 {
                  tunnel: w545 -> [_ w565]
                  tunnel: w544 -> [_ w564]
                  tunnel: [_ w563] -> w540
                  frame Default {
                  }
                  frame "Sideband" {
                    n221 = Format Value(string ("")="s=", format string=w565, value (0)=w564) -> (output string=w563:string)
                  }
                }
                n222 = case shown="True" w541 {
                  tunnel: w543 -> [w556 w560]
                  tunnel: [w556 w562] -> w542
                  tunnel: w540 -> [_ w558]
                  frame False {
                  }
                  frame True {
                    n223 = Matrix Size(0:w560) -> (1:w561:i32)  [unwired: 1 out]
                    n224 = Decrement(x=w561) -> (x-1=w559:i32)
                    n225 = Replace Array Subset(array=w560, new element=w558, index (row)=w559, index (col)=0 ("disabled index (col)")) -> (w562:string[][])
                  }
                }
                n226 = for {
                  tunnel: w549 -> [w569] mode=indexing
                  tunnel: [w568] -> w551 mode=indexing
                  tunnel: w550 -> [w567]
                  n227 = Format Value(format string=w567, value (0)=w569) -> (output string=w568:string)  [unwired: 1 in]
                }
                n228 = Build Array (concatenate)(w546, w551) -> (w548:string[])
                n229 = Build Array (concatenate)(w555, w554) -> (w553:string[])
                n230 = Build Array (concatenate)(w542, w548) -> (w552:string[][])
              }
              frame "XY" {
                n231 = Get Variant Attribute(Variant=w585, name="xy type", default value (empty Variant)=u16 0 ("precision (6)")) -> (duplicate Variant=w584:variant, value=w581:u16)  [unwired: 1 in, 2 out]
                n232 = case shown="1" w581 {
                  tunnel: [0.0 ("element") w606] -> w578
                  tunnel: w584 -> [_ w609]
                  tunnel: w575 -> [_ w607]
                  tunnel: [_ w605] -> w571
                  frame 0, Default {
                  }
                  frame 1 {
                    n233 = Get Variant Attribute(Variant=w609, name="y reference", default value (empty Variant)=0.0 ("element")) -> (value=w606:dbl)  [unwired: 1 in, 3 out]
                    n234 = Format Value(string ("")="ref=", format string=w607, value (0)=w606) -> (output string=w605:string)
                  }
                }
                n235 = case shown="True" w574 {
                  tunnel: w573 -> [w591 w596]
                  tunnel: [w591 w600] -> w572
                  tunnel: w571 -> [_ w599]
                  tunnel: w570 -> [_ w598]
                  frame False {
                  }
                  frame True {
                    n236 = Initialize Array(w599, w598) -> (w594:string[])
                    n237 = Matrix Size(0:w596) -> (1:w597:i32)  [unwired: 1 out]
                    n238 = Build Array (concatenate)("", w594) -> (w592:string[])
                    n239 = Decrement(x=w597) -> (x-1=w595:i32)
                    n240 = Replace Array Subset(array=w596, new element=w592, index (row)=w595) -> (w600:string[][])  [unwired: 1 in]
                  }
                }
                n241 = Subtract(x=w586, y=w578) -> (x-y=w577:dbl[])
                n242 = for {
                  tunnel: w577 -> [w603] mode=indexing
                  tunnel: [w602] -> w576 mode=indexing
                  tunnel: w575 -> [w601]
                  n243 = Format Value(format string=w601, value (0)=w603) -> (output string=w602:string)  [unwired: 1 in]
                }
                n244 = Build Array (concatenate)(w580, w576) -> (w579:string[])
                n245 = Build Array (concatenate)(w590, w589) -> (w588:string[])
                n246 = Build Array (concatenate)(w572, w579) -> (w587:string[][])
              }
              frame "Band", "Differential", "Integral", "Pair" {
                n247 = for {
                  tunnel: w624 -> [w684] mode=indexing
                  tunnel: [w683] -> w627 mode=indexing
                  tunnel: w614 -> [w682]
                  n248 = Format Value(format string=w682, value (0)=w684) -> (output string=w683:string)  [unwired: 1 in]
                }
                n249 = Index Array(array=w618) -> (element=w617:dbl)  [unwired: 1 in]
                n250 = Build Array (concatenate)(w626, w627) -> (w625:string[])
                n251 = Build Array (concatenate)(w617, w624) -> (w616:dbl[])
                n252 = Build Array (concatenate)(w629, w623) -> (w621:string[])
                n253 = Build Array (concatenate)(w628, w625) -> (w620:string[][])
                n254 = feedback-in #6(w616) -> ()
                n255 = feedback #6() -> (w615:dbl[])  [unwired: 1 in]
                n256 = case shown="\"B2\"" w623 {
                  tunnel: [w631 w681] -> w622
                  tunnel: w621 -> [w653 w681]
                  tunnel: w620 -> [w651 w680]
                  tunnel: [w630 w680] -> w619
                  tunnel: w616 -> [w638 _]
                  tunnel: w615 -> [w640 _]
                  tunnel: w614 -> [w649 _]
                  tunnel: w613 -> [w643 _]
                  tunnel: w612 -> [w642 _]
                  frame "B2" {
                    n257 = Subtract(x=w638, y=w640) -> (x-y=w647:dbl[])
                    n258 = Index Array(array=w640) -> (element=w639:dbl)  [unwired: 1 in]
                    n259 = Index Array(array=w638) -> (element=w637:dbl)  [unwired: 1 in]
                    n260 = Index Array(array=w647) -> (element=w648:dbl)  [unwired: 1 in]
                    n261 = Bundle By Name(cluster=cluster{"start":dbl, "stop":dbl} {"start"=-1.0, "stop"=-1.0} ("range"), "start"=w639, "stop"=w637) -> (w641:cluster{"start":dbl, "stop":dbl})
                    n262 = Divide(x=w647, y=w648) -> (x/y=w646:dbl[])
                    n263 = call-poly <vilib>:"SVFA Get Spectrum Subset.vi"("spectra"=w643, "range"=w641, "spectrum info"=w642) -> ("spectra subsets"=w636:cluster{"x0":dbl, "dx":dbl, "magnitude":dbl[]}[], "actual ranges"=w633:cluster{"start":dbl, "stop":dbl}[])  [unwired: 11 in, 4 out]
                    n264 = for {
                      tunnel: w647 -> [w662] mode=indexing
                      tunnel: [w661] -> w650 mode=indexing
                      tunnel: w649 -> [w656]
                      tunnel: w646 -> [w660] mode=indexing
                      tunnel: [w659] -> w645 mode=indexing
                      tunnel: w636 -> [w657]
                      tunnel: [w655] -> w635 mode=indexing
                      tunnel: w633 -> [w654]
                      i -> [w658]
                      n265 = case shown="Default" w658 {
                        selector: w658 -> [_ w679]
                        tunnel: w657 -> [_ w678]
                        tunnel: w656 -> [w665 w677]
                        tunnel: [w664 w676] -> w655
                        tunnel: w654 -> [w671 _]
                        frame 0 {
                          n266 = Index Array(array=w671) -> (element=w663:cluster{"start":dbl, "stop":dbl})  [unwired: 1 in]
                          n267 = Unbundle(w663) -> ("start"=w670:dbl, "stop"=w669:dbl)
                          n268 = Compound Arithmetic op=ADD(w670, w669) -> (w668:dbl)
                          n269 = Compound Arithmetic op=MULTIPLY(w668, 0.5 ("value")) -> (w666:dbl)
                          n270 = Format Value(format string=w665, value (0)=w666) -> (output string=w664:string)  [unwired: 1 in]
                        }
                        frame Default {
                          n271 = Decrement(x=w679) -> (x-1=w672:i32)
                          n272 = Index Array(array=w678, index=w672) -> (element=w675:cluster{"x0":dbl, "dx":dbl, "magnitude":dbl[]})
                          n273 = Unbundle(w675) -> ("magnitude"=w674:dbl[])  [unwired: 2 out]
                          n274 = call-poly <vilib>:"Mean.vi"("X"=w674) -> ("mean"=w673:dbl)  [unwired: 1 out]
                          n275 = Format Value(format string=w677, value (0)=w673) -> (output string=w676:string)  [unwired: 1 in]
                        }
                      }
                      n276 = Format Value(format string=w656, value (0)=w662) -> (output string=w661:string)  [unwired: 1 in]
                      n277 = Format Value(format string=w656, value (0)=w660) -> (output string=w659:string)  [unwired: 1 in]
                    }
                    n278 = Build Array (concatenate)(w653, "b2-b1", "dy/dx", "average in band") -> (w631:string[])
                    n279 = Build Array (concatenate)(w651, w650, w645, w635) -> (w630:string[][])
                  }
                  frame "B1", Default {
                  }
                }
              }
            }
          }
        }
        frame 36 {
          w738 = "" ("String")
          w708 = "" ("String")
          n280 = Unbundle By Name(w700) -> ("X Scale.Format String"=w702:string)
          n281 = for {
            tunnel: w753 -> [w785] mode=indexing
            tunnel: [w773] -> w685 mode=indexing
            tunnel: w725 -> [w786] mode=indexing
            tunnel: ["" ("String")] -> w748 mode=indexing
            tunnel: w752 -> [w782]
            tunnel: w751 -> [w779]
            tunnel: [w778] -> w688 mode=indexing
            tunnel: [w776] -> w689 mode=indexing
            tunnel: [w775] -> w712 mode=indexing
            tunnel: [w774] -> w749
            tunnel: w702 -> [w771]
            tunnel: [w772] -> w718 mode=indexing
            tunnel: [w770] -> w705 mode=indexing
            workers-P: _ -> [_]
            # "For each channel"
            n282 = call <vilib>:"svc_Spectrum Units.vi"("spectrum info in"=w785) -> ("x-axis unit label"=w774:string, "spectrum info out"=w784:T6)  [unwired: 3 in, 2 out]
            n283 = Unbundle By Name(w786) -> ("dx"=w772:dbl)
            n284 = Unbundle By Name(w784) -> ("channel name"=w773:string, "spectral info.window"=w781:u16)
            n285 = call <vilib>:"svfa_Spectrum Info Window to windowTd Type Def.vi"("window"=w781) -> ("window"=w770:T13)  [unwired: 4 in]
            n286 = call <vilib>:"svc_Window Parameters.vi"("window"=w770) -> ("6dB BW"=w783:dbl)  [unwired: 7 in, 3 out]
            n287 = Search 1D Array(1D array=w782, element=w770) -> (index of element=w780:i32)  [unwired: 1 in]
            n288 = Multiply(x=w772, y=w783) -> (x*y=w777:dbl)
            n289 = case shown="Default" w780 {
              selector: w780 -> [_ w790]
              tunnel: w779 -> [_ w789]
              tunnel: ["" ("String") w788] -> w775
              frame ..-1 {
              }
              frame Default {
                n290 = Index Array(array=w789, index=w790) -> (element=w788:string)
              }
            }
            n291 = Format Into String(format string=w771, w772) -> (resulting string=w778:string)  [unwired: 2 in, 1 out]
            n292 = Format Into String(format string=w771, w777) -> (resulting string=w776:string)  [unwired: 2 in, 1 out]
          }
          n293 = Unbundle By Name(w697) -> ("Controls.Graph"=w704:refnum<vi>)
          n294 = feedback #7() -> (w687:string[])  [unwired: 1 in]
          n295 = feedback-in #7(w685) -> ()
          n296 = Array Max & Min(array=w718) -> (min value=w719:dbl, min index (indices)=w723:i32)  [unwired: 2 out]
          n297 = Array Max & Min(array=w705) -> (min value=w722:T13, min index (indices)=w715:i32)  [unwired: 2 out]
          n298 = Not Equal?(x=w685, y=w687) -> (x != y?=w686:bool)
          n299 = Equal?(x=w719, y=w718) -> (x = y?=w720:bool[])
          n300 = Equal?(x=w705, y=w722) -> (x = y?=w721:bool[])
          n301 = Bundle By Name(cluster=w700, "X Increment"=w719) -> (w699:T2)
          n302 = And Array Elements(Boolean array=w720) -> (logical AND=w709:bool)
          n303 = And Array Elements(Boolean array=w721) -> (logical AND=w711:bool)
          n304 = case shown="True" w686 {
            tunnel: w704 -> [w755 w758]
            tunnel: [w755 w757] -> w694
            tunnel: w685 -> [_ w756]
            frame False {
            }
            frame True {
              n305 = for {
                tunnel: w758 -> [w762]
                tunnel: w756 -> [w760] mode=indexing
                tunnel: [w759] -> w757
                i -> [w761]
                n306 = property class="WFGraph (strict)"(reference=w762, "Active Plot"=w761, "Plot.Plot Name"=w760) -> (reference out=w759:refnum<vi>)  [unwired: 1 in, 1 out]
              }
            }
          }
          n307 = And(x=w709, y=w711) -> (x .and. y?=w716:bool)
          n308 = Index Array(array=w688, index=w723) -> (element=w707:string)
          n309 = Index Array(array=w689, index=w715) -> (element=w717:string)
          n310 = Index Array(array=w712, index=w715) -> (element=w713:string)
          n311 = feedback #8() -> (w724:i32)  [unwired: 1 in]
          n312 = feedback-in #8(w693) -> ()
          n313 = Select(t=w707, s=w709, f=w708) -> (s? t:f=w706:string)
          n314 = Select(t=w717, s=w716, f=w708) -> (s? t:f=w714:string)
          n315 = Select(t=w713, s=w711, f=w708) -> (s? t:f=w710:string)
          n316 = Index Array(array=w725) -> (element=w733:cluster{"x0":dbl, "dx":dbl, "Y":dbl[]})  [unwired: 1 in]
          n317 = Not Equal?(x=w693, y=w724) -> (x != y?=w695:bool)
          n318 = case shown="True" w695 {
            tunnel: w699 -> [w764 w768]
            tunnel: [w764 w767] -> w698
            tunnel: w697 -> [w763 w766]
            tunnel: [w763 w766] -> w696
            tunnel: w693 -> [_ w765]
            tunnel: w694 -> [_ _]
            frame False {
            }
            frame True {
              n319 = call <vilib>:"Resize and Align.vi"("number of channels"=w765, "Refnums for Resizing and Alignment"=w766, "State in"=w768) -> ("State out"=w767:T2)  [unwired: 7 in, 1 out]
            }
          }
          n320 = Build Array (concatenate)("X" ("String"), w685) -> (w739:string[])
          n321 = Build Array (concatenate)(w706, w688) -> (w743:string[])
          n322 = Build Array (concatenate)(w714, w689) -> (w746:string[])
          n323 = Build Array (concatenate)(w710, w712) -> (w742:string[])
          n324 = Build Array (concatenate)(w749, w748) -> (w747:string[])
          n325 = Unbundle By Name(w733) -> ("x0"=w726:dbl, "dx"=w729:dbl, "Y"=w732:dbl[])
          n326 = Array Size(array=w732) -> (size(s)=w731:i32)
          n327 = Build Array(w743, w746, w742, w747) -> (w736:string[][])
          n328 = Unbundle By Name(w698) -> ("X Scale.Format String"=w701:string, "Cursors"=w692:T14)
          n329 = Unbundle By Name(w696) -> ("Controls.Table"=w703:refnum<vi>)
          n330 = Decrement(x=w731) -> (x-1=w730:i32)
          n331 = Multiply(x=w729, y=w730) -> (x*y=w728:dbl)
          n332 = Array Size(array=w725) -> (size(s)=w735:i32)
          n333 = Add(x=w726, y=w728) -> (x+y=w727:dbl)
          n334 = Unbundle By Name(w692) -> ("List"=w691:T15, "Tags"=w690:variant[])
          n335 = Unbundle By Name(w698) -> ("Y Scale.Format String"=w737:string, "Measurement Cursor Configuration.sideband.X spacing (s)"=w734:dbl)
          n336 = for {
            tunnel: w725 -> [w801]
            tunnel: w753 -> [w800]
            tunnel: T12."coerce to nearest" ("frequency coercion") -> [w826]
            shift-right: [w824] -> w740
            shift-left: string[] ["dx", "RBW", "Window", "Units"] ("Array") -> [w816]
            shift-right: [w823] -> w741
            shift-left: w736 -> [w817]
            tunnel: "cursor type" -> [w822]
            shift-right: [w791] -> _
            shift-left: w738 -> [w821]
            tunnel: w738 -> [w820]
            tunnel: w701 -> [w792]
            tunnel: w737 -> [w806]
            tunnel: w735 -> [w804]
            tunnel: w734 -> [w803]
            tunnel: w727 -> [w798]
            tunnel: w726 -> [w797]
            tunnel: w691 -> [w796] mode=indexing
            tunnel: w690 -> [w793] mode=indexing
            # "format for display = first letter capitalization"
            # "For each cursor"
            n337 = Unbundle By Name(w796) -> ("Name"=w795:string, "Position.X"=w794:dbl)
            n338 = Get Variant Attribute(Variant=w793, name=w822, default value (empty Variant)=w820) -> (duplicate Variant=w808:variant, value=w809:string)  [unwired: 1 in, 2 out]
            n339 = Search/Split String(string=w809, offset (0)=1) -> (substring before match=w812:string, match + rest of string=w810:string)  [unwired: 1 in, 1 out]
            n340 = To Upper Case(1:w812) -> (0:w811:string)
            n341 = Concatenate Strings(w811, w810) -> (w791:string)
            n342 = Not Equal?(x=w821, y=w791) -> (x != y?=w819:bool)
            n343 = case shown="\"Band\", \"Differential\", \"Integral\", \"Pair\"" w791 {
              tunnel: w794 -> [w827 w831]
              tunnel: [w827 w830] -> w799
              tunnel: w798 -> [_ w829]
              tunnel: w797 -> [_ w828]
              frame Default {
              }
              frame "Band", "Differential", "Integral", "Pair" {
                n344 = In Range and Coerce(upper limit=w828, x=w831, lower limit=w829) -> (coerced(x)=w830:dbl)  [unwired: 1 out]
              }
            }
            n345 = case shown="True" w819 {
              selector: w819 -> [w832 w836]
              tunnel: [w835 w844] -> w818
              tunnel: w795 -> [w835 w844]
              tunnel: w817 -> [w833 w839]
              tunnel: w816 -> [w834 w842]
              tunnel: [w834 w843] -> w815
              tunnel: [w833 w840] -> w814
              tunnel: w791 -> [_ w841]
              tunnel: [w832 w836] -> w805
              frame False {
              }
              frame True {
                # "new section in table\n--> add header row"
                n346 = Build Array("") -> (w837:string[])
                n347 = Build Array (concatenate)(w842, w841) -> (w843:string[])
                n348 = Build Array (concatenate)(w839, w837) -> (w840:string[][])
              }
            }
            n349 = Format Into String(format string=w792, w799) -> (resulting string=w807:string)  [unwired: 2 in, 1 out]
            n350 = call-poly <vilib>:"SVFA Get Spectrum Value.vi"("spectra"=w801, "x value (1000)"=w799, "coercion (nearest)"=w826, "spectrum info"=w800) -> ("spectra values"=w825:dbl[], "actual x values"=w802:dbl[])  [unwired: 11 in, 3 out]
            n351 = case shown="\"Band\", \"Differential\", \"Integral\", \"Pair\"" w791 {
              selector: w791 -> [w852 _ _]
              tunnel: w825 -> [w854 w891 w929]
              tunnel: w815 -> [w860 w895 w934]
              tunnel: w818 -> [w859 w894 w928]
              tunnel: [w858 w893 w927] -> w824
              tunnel: w814 -> [w848 w878 w933]
              tunnel: [w857 w892 w924] -> w823
              tunnel: w808 -> [_ w890 _]
              tunnel: w807 -> [w851 w885 w931]
              tunnel: w806 -> [w855 w880 w919]
              tunnel: w805 -> [w846 w879 _]
              tunnel: w804 -> [_ w875 _]
              tunnel: w792 -> [w850 _ _]
              tunnel: w803 -> [w849 _ _]
              tunnel: w802 -> [_ _ w923]
              tunnel: w801 -> [_ _ w918]
              tunnel: w800 -> [_ _ w917]
              frame Default {
                n352 = case shown="\"Sideband\"" w852 {
                  tunnel: w850 -> [_ w870]
                  tunnel: w849 -> [_ w869]
                  tunnel: [_ w868] -> w845
                  frame Default {
                  }
                  frame "Sideband" {
                    n353 = Format Value(string ("")="s=", format string=w870, value (0)=w869) -> (output string=w868:string)
                  }
                }
                n354 = case shown="True" w846 {
                  tunnel: w848 -> [w861 w865]
                  tunnel: [w861 w867] -> w847
                  tunnel: w845 -> [_ w863]
                  frame False {
                  }
                  frame True {
                    n355 = Matrix Size(0:w865) -> (1:w866:i32)  [unwired: 1 out]
                    n356 = Decrement(x=w866) -> (x-1=w864:i32)
                    n357 = Replace Array Subset(array=w865, new element=w863, index (row)=w864, index (col)=0 ("disabled index (col)")) -> (w867:string[][])
                  }
                }
                n358 = for {
                  tunnel: w854 -> [w874] mode=indexing
                  tunnel: [w873] -> w856 mode=indexing
                  tunnel: w855 -> [w872]
                  n359 = Format Value(format string=w872, value (0)=w874) -> (output string=w873:string)  [unwired: 1 in]
                }
                n360 = Build Array (concatenate)(w851, w856) -> (w853:string[])
                n361 = Build Array (concatenate)(w860, w859) -> (w858:string[])
                n362 = Build Array (concatenate)(w847, w853) -> (w857:string[][])
              }
              frame "XY" {
                n363 = Get Variant Attribute(Variant=w890, name="xy type", default value (empty Variant)=u16 0 ("precision (6)")) -> (duplicate Variant=w889:variant, value=w886:u16)  [unwired: 1 in, 2 out]
                n364 = case shown="1" w886 {
                  tunnel: [0.0 ("element") w911] -> w883
                  tunnel: w889 -> [_ w914]
                  tunnel: w880 -> [_ w912]
                  tunnel: [_ w910] -> w876
                  frame 0, Default {
                  }
                  frame 1 {
                    n365 = Get Variant Attribute(Variant=w914, name="y reference", default value (empty Variant)=0.0 ("element")) -> (value=w911:dbl)  [unwired: 1 in, 3 out]
                    n366 = Format Value(string ("")="ref=", format string=w912, value (0)=w911) -> (output string=w910:string)
                  }
                }
                n367 = case shown="True" w879 {
                  tunnel: w878 -> [w896 w901]
                  tunnel: [w896 w905] -> w877
                  tunnel: w876 -> [_ w904]
                  tunnel: w875 -> [_ w903]
                  frame False {
                  }
                  frame True {
                    n368 = Initialize Array(w904, w903) -> (w899:string[])
                    n369 = Matrix Size(0:w901) -> (1:w902:i32)  [unwired: 1 out]
                    n370 = Build Array (concatenate)("", w899) -> (w897:string[])
                    n371 = Decrement(x=w902) -> (x-1=w900:i32)
                    n372 = Replace Array Subset(array=w901, new element=w897, index (row)=w900) -> (w905:string[][])  [unwired: 1 in]
                  }
                }
                n373 = Subtract(x=w891, y=w883) -> (x-y=w882:dbl[])
                n374 = for {
                  tunnel: w882 -> [w908] mode=indexing
                  tunnel: [w907] -> w881 mode=indexing
                  tunnel: w880 -> [w906]
                  n375 = Format Value(format string=w906, value (0)=w908) -> (output string=w907:string)  [unwired: 1 in]
                }
                n376 = Build Array (concatenate)(w885, w881) -> (w884:string[])
                n377 = Build Array (concatenate)(w895, w894) -> (w893:string[])
                n378 = Build Array (concatenate)(w877, w884) -> (w892:string[][])
              }
              frame "Band", "Differential", "Integral", "Pair" {
                n379 = for {
                  tunnel: w929 -> [w989] mode=indexing
                  tunnel: [w988] -> w932 mode=indexing
                  tunnel: w919 -> [w987]
                  n380 = Format Value(format string=w987, value (0)=w989) -> (output string=w988:string)  [unwired: 1 in]
                }
                n381 = Index Array(array=w923) -> (element=w922:dbl)  [unwired: 1 in]
                n382 = Build Array (concatenate)(w931, w932) -> (w930:string[])
                n383 = Build Array (concatenate)(w922, w929) -> (w921:dbl[])
                n384 = Build Array (concatenate)(w934, w928) -> (w926:string[])
                n385 = Build Array (concatenate)(w933, w930) -> (w925:string[][])
                n386 = feedback-in #9(w921) -> ()
                n387 = feedback #9() -> (w920:dbl[])  [unwired: 1 in]
                n388 = case shown="\"B2\"" w928 {
                  tunnel: [w936 w986] -> w927
                  tunnel: w926 -> [w958 w986]
                  tunnel: w925 -> [w956 w985]
                  tunnel: [w935 w985] -> w924
                  tunnel: w921 -> [w943 _]
                  tunnel: w920 -> [w945 _]
                  tunnel: w919 -> [w954 _]
                  tunnel: w918 -> [w948 _]
                  tunnel: w917 -> [w947 _]
                  frame "B2" {
                    n389 = Subtract(x=w943, y=w945) -> (x-y=w952:dbl[])
                    n390 = Index Array(array=w945) -> (element=w944:dbl)  [unwired: 1 in]
                    n391 = Index Array(array=w943) -> (element=w942:dbl)  [unwired: 1 in]
                    n392 = Index Array(array=w952) -> (element=w953:dbl)  [unwired: 1 in]
                    n393 = Bundle By Name(cluster=cluster{"start":dbl, "stop":dbl} {"start"=-1.0, "stop"=-1.0} ("range"), "start"=w944, "stop"=w942) -> (w946:cluster{"start":dbl, "stop":dbl})
                    n394 = Divide(x=w952, y=w953) -> (x/y=w951:dbl[])
                    n395 = call-poly <vilib>:"SVFA Get Spectrum Subset.vi"("spectra"=w948, "range"=w946, "spectrum info"=w947) -> ("spectra subsets"=w941:cluster{"x0":dbl, "dx":dbl, "magnitude":dbl[]}[], "actual ranges"=w938:cluster{"start":dbl, "stop":dbl}[])  [unwired: 11 in, 4 out]
                    n396 = for {
                      tunnel: w952 -> [w967] mode=indexing
                      tunnel: [w966] -> w955 mode=indexing
                      tunnel: w954 -> [w961]
                      tunnel: w951 -> [w965] mode=indexing
                      tunnel: [w964] -> w950 mode=indexing
                      tunnel: w941 -> [w962]
                      tunnel: [w960] -> w940 mode=indexing
                      tunnel: w938 -> [w959]
                      i -> [w963]
                      n397 = case shown="Default" w963 {
                        selector: w963 -> [_ w984]
                        tunnel: w962 -> [_ w983]
                        tunnel: w961 -> [w970 w982]
                        tunnel: [w969 w981] -> w960
                        tunnel: w959 -> [w976 _]
                        frame 0 {
                          n398 = Index Array(array=w976) -> (element=w968:cluster{"start":dbl, "stop":dbl})  [unwired: 1 in]
                          n399 = Unbundle(w968) -> ("start"=w975:dbl, "stop"=w974:dbl)
                          n400 = Compound Arithmetic op=ADD(w975, w974) -> (w973:dbl)
                          n401 = Compound Arithmetic op=MULTIPLY(w973, 0.5 ("value")) -> (w971:dbl)
                          n402 = Format Value(format string=w970, value (0)=w971) -> (output string=w969:string)  [unwired: 1 in]
                        }
                        frame Default {
                          n403 = Decrement(x=w984) -> (x-1=w977:i32)
                          n404 = Index Array(array=w983, index=w977) -> (element=w980:cluster{"x0":dbl, "dx":dbl, "magnitude":dbl[]})
                          n405 = Unbundle(w980) -> ("magnitude"=w979:dbl[])  [unwired: 2 out]
                          n406 = call-poly <vilib>:"Mean.vi"("X"=w979) -> ("mean"=w978:dbl)  [unwired: 1 out]
                          n407 = Format Value(format string=w982, value (0)=w978) -> (output string=w981:string)  [unwired: 1 in]
                        }
                      }
                      n408 = Format Value(format string=w961, value (0)=w967) -> (output string=w966:string)  [unwired: 1 in]
                      n409 = Format Value(format string=w961, value (0)=w965) -> (output string=w964:string)  [unwired: 1 in]
                    }
                    n410 = Build Array (concatenate)(w958, "b2-b1", "dy/dx", "average in band") -> (w936:string[])
                    n411 = Build Array (concatenate)(w956, w955, w950, w940) -> (w935:string[][])
                  }
                  frame "B1", Default {
                  }
                }
              }
            }
          }
        }
        frame 34, 35 {
          w1046 = "" ("String")
          w1013 = "" ("String")
          n412 = Unbundle By Name(w1005) -> ("X Scale.Format String"=w1007:string)
          n413 = for {
            tunnel: w1061 -> [w1103] mode=indexing
            tunnel: [w1080] -> w990 mode=indexing
            tunnel: w1031 -> [w1104] mode=indexing
            tunnel: [w1084] -> w1056 mode=indexing
            tunnel: w1060 -> [w1100]
            tunnel: w1059 -> [w1097]
            tunnel: [w1096] -> w993 mode=indexing
            tunnel: [w1094] -> w994 mode=indexing
            tunnel: [w1093] -> w1017 mode=indexing
            tunnel: [w1092] -> w1057
            tunnel: [w1082] -> w1044 mode=indexing
            tunnel: w1007 -> [w1078]
            tunnel: [w1079] -> w1023 mode=indexing
            tunnel: [w1077] -> w1010 mode=indexing
            workers-P: _ -> [_]
            # "For each channel"
            n414 = call <vilib>:"svc_Spectrum Units.vi"("spectrum info in"=w1103) -> ("x-axis unit label"=w1092:string, "spectrum info out"=w1102:T6, "unit label"=w1083:string)  [unwired: 3 in, 1 out]
            n415 = Unbundle By Name(w1102) -> ("channel name"=w1080:string, "spectral info.window"=w1099:u16, "dB reference [EU]"=w1090:dbl)
            n416 = Unbundle By Name(w1104) -> ("dx"=w1079:dbl)
            n417 = call <vilib>:"svfa_Spectrum Info Window to windowTd Type Def.vi"("window"=w1099) -> ("window"=w1077:T13)  [unwired: 4 in]
            n418 = Number To Engineering String(2:i16 2 ("precision (6)"), 4:w1090) -> (0:w1081:string)  [unwired: 2 in]
            n419 = Match Pattern(string=w1083, regular expression=" ref ") -> (before substring=w1087:string, match substring=w1086:string, after substring=w1085:string, offset past match=w1088:i32)  [unwired: 1 in]
            n420 = call <vilib>:"svc_Window Parameters.vi"("window"=w1077) -> ("6dB BW"=w1101:dbl)  [unwired: 7 in, 3 out]
            n421 = Search 1D Array(1D array=w1100, element=w1077) -> (index of element=w1098:i32)  [unwired: 1 in]
            n422 = case shown="-1" w1088 {
              tunnel: w1087 -> [_ w1108]
              tunnel: w1086 -> [_ _]
              tunnel: w1085 -> [_ w1107]
              tunnel: [w1106 w1108] -> w1084
              tunnel: w1083 -> [w1106 _]
              tunnel: [w1105 w1107] -> w1082
              tunnel: w1081 -> [w1105 _]
              frame -1 {
              }
              frame Default {
              }
            }
            n423 = Multiply(x=w1079, y=w1101) -> (x*y=w1095:dbl)
            n424 = case shown="Default" w1098 {
              selector: w1098 -> [_ w1112]
              tunnel: w1097 -> [_ w1111]
              tunnel: ["" ("String") w1110] -> w1093
              frame ..-1 {
              }
              frame Default {
                n425 = Index Array(array=w1111, index=w1112) -> (element=w1110:string)
              }
            }
            n426 = Format Into String(format string=w1078, w1079) -> (resulting string=w1096:string)  [unwired: 2 in, 1 out]
            n427 = Format Into String(format string=w1078, w1095) -> (resulting string=w1094:string)  [unwired: 2 in, 1 out]
          }
          n428 = Unbundle By Name(w1002) -> ("Controls.Graph"=w1009:refnum<vi>)
          n429 = feedback #10() -> (w992:string[])  [unwired: 1 in]
          n430 = feedback-in #10(w990) -> ()
          n431 = Array Max & Min(array=w1023) -> (min value=w1024:dbl, min index (indices)=w1029:i32)  [unwired: 2 out]
          n432 = Array Max & Min(array=w1010) -> (min value=w1027:T13, min index (indices)=w1020:i32)  [unwired: 2 out]
          n433 = Not Equal?(x=w990, y=w992) -> (x != y?=w991:bool)
          n434 = Equal?(x=w1024, y=w1023) -> (x = y?=w1025:bool[])
          n435 = Equal?(x=w1010, y=w1027) -> (x = y?=w1026:bool[])
          n436 = Bundle By Name(cluster=w1005, "X Increment"=w1024) -> (w1004:T2)
          n437 = And Array Elements(Boolean array=w1025) -> (logical AND=w1014:bool)
          n438 = And Array Elements(Boolean array=w1026) -> (logical AND=w1016:bool)
          n439 = case shown="True" w991 {
            tunnel: w1009 -> [w1063 w1066]
            tunnel: [w1063 w1065] -> w999
            tunnel: w990 -> [_ w1064]
            frame False {
            }
            frame True {
              n440 = for {
                tunnel: w1066 -> [w1070]
                tunnel: w1064 -> [w1068] mode=indexing
                tunnel: [w1067] -> w1065
                i -> [w1069]
                n441 = property class="WFGraph (strict)"(reference=w1070, "Active Plot"=w1069, "Plot.Plot Name"=w1068) -> (reference out=w1067:refnum<vi>)  [unwired: 1 in, 1 out]
              }
            }
          }
          n442 = And(x=w1014, y=w1016) -> (x .and. y?=w1021:bool)
          n443 = Index Array(array=w993, index=w1029) -> (element=w1012:string)
          n444 = Index Array(array=w994, index=w1020) -> (element=w1022:string)
          n445 = Index Array(array=w1017, index=w1020) -> (element=w1018:string)
          n446 = feedback #11() -> (w1030:i32)  [unwired: 1 in]
          n447 = feedback-in #11(w998) -> ()
          n448 = Select(t=w1012, s=w1014, f=w1013) -> (s? t:f=w1011:string)
          n449 = Select(t=w1022, s=w1021, f=w1013) -> (s? t:f=w1019:string)
          n450 = Select(t=w1018, s=w1016, f=w1013) -> (s? t:f=w1015:string)
          n451 = Index Array(array=w1031) -> (element=w1039:cluster{"x0":dbl, "dx":dbl, "Y":dbl[]})  [unwired: 1 in]
          n452 = Not Equal?(x=w998, y=w1030) -> (x != y?=w1000:bool)
          n453 = case shown="True" w1000 {
            tunnel: w1004 -> [w1072 w1076]
            tunnel: [w1072 w1075] -> w1003
            tunnel: w1002 -> [w1071 w1074]
            tunnel: [w1071 w1074] -> w1001
            tunnel: w998 -> [_ w1073]
            tunnel: w999 -> [_ _]
            frame False {
            }
            frame True {
              n454 = call <vilib>:"Resize and Align.vi"("number of channels"=w1073, "Refnums for Resizing and Alignment"=w1074, "State in"=w1076) -> ("State out"=w1075:T2)  [unwired: 7 in, 1 out]
            }
          }
          n455 = Build Array (concatenate)("X" ("String"), w990) -> (w1047:string[])
          n456 = Build Array (concatenate)(w1011, w993) -> (w1051:string[])
          n457 = Build Array (concatenate)(w1019, w994) -> (w1054:string[])
          n458 = Build Array (concatenate)(w1015, w1017) -> (w1050:string[])
          n459 = Build Array (concatenate)(w1057, w1056) -> (w1055:string[])
          n460 = Build Array (concatenate)("1.0" ("String"), w1044) -> (w1045:string[])
          n461 = Unbundle By Name(w1039) -> ("x0"=w1032:dbl, "dx"=w1035:dbl, "Y"=w1038:dbl[])
          n462 = Array Size(array=w1038) -> (size(s)=w1037:i32)
          n463 = Build Array(w1051, w1054, w1050, w1055, w1045) -> (w1042:string[][])
          n464 = Unbundle By Name(w1003) -> ("X Scale.Format String"=w1006:string, "Cursors"=w997:T14)
          n465 = Unbundle By Name(w1001) -> ("Controls.Table"=w1008:refnum<vi>)
          n466 = Decrement(x=w1037) -> (x-1=w1036:i32)
          n467 = Multiply(x=w1035, y=w1036) -> (x*y=w1034:dbl)
          n468 = Array Size(array=w1031) -> (size(s)=w1041:i32)
          n469 = Add(x=w1032, y=w1034) -> (x+y=w1033:dbl)
          n470 = Unbundle By Name(w997) -> ("List"=w996:T15, "Tags"=w995:variant[])
          n471 = Unbundle By Name(w1003) -> ("Y Scale.Format String"=w1043:string, "Measurement Cursor Configuration.sideband.X spacing (s)"=w1040:dbl)
          n472 = for {
            tunnel: w1031 -> [w1123]
            tunnel: w1061 -> [w1122]
            tunnel: T12."coerce to nearest" ("frequency coercion") -> [w1148]
            shift-right: [w1146] -> w1048
            shift-left: string[] ["dx", "RBW", "Window", "Units", "Reference"] ("Array") -> [w1138]
            shift-right: [w1145] -> w1049
            shift-left: w1042 -> [w1139]
            tunnel: "cursor type" -> [w1144]
            shift-right: [w1113] -> _
            shift-left: w1046 -> [w1143]
            tunnel: w1046 -> [w1142]
            tunnel: w1006 -> [w1114]
            tunnel: w1043 -> [w1128]
            tunnel: w1041 -> [w1126]
            tunnel: w1040 -> [w1125]
            tunnel: w1033 -> [w1120]
            tunnel: w1032 -> [w1119]
            tunnel: w996 -> [w1118] mode=indexing
            tunnel: w995 -> [w1115] mode=indexing
            # "format for display = first letter capitalization"
            # "For each cursor"
            n473 = Unbundle By Name(w1118) -> ("Name"=w1117:string, "Position.X"=w1116:dbl)
            n474 = Get Variant Attribute(Variant=w1115, name=w1144, default value (empty Variant)=w1142) -> (duplicate Variant=w1130:variant, value=w1131:string)  [unwired: 1 in, 2 out]
            n475 = Search/Split String(string=w1131, offset (0)=1) -> (substring before match=w1134:string, match + rest of string=w1132:string)  [unwired: 1 in, 1 out]
            n476 = To Upper Case(1:w1134) -> (0:w1133:string)
            n477 = Concatenate Strings(w1133, w1132) -> (w1113:string)
            n478 = Not Equal?(x=w1143, y=w1113) -> (x != y?=w1141:bool)
            n479 = case shown="\"Band\", \"Differential\", \"Integral\", \"Pair\"" w1113 {
              tunnel: w1116 -> [w1149 w1153]
              tunnel: [w1149 w1152] -> w1121
              tunnel: w1120 -> [_ w1151]
              tunnel: w1119 -> [_ w1150]
              frame Default {
              }
              frame "Band", "Differential", "Integral", "Pair" {
                n480 = In Range and Coerce(upper limit=w1150, x=w1153, lower limit=w1151) -> (coerced(x)=w1152:dbl)  [unwired: 1 out]
              }
            }
            n481 = case shown="True" w1141 {
              selector: w1141 -> [w1154 w1158]
              tunnel: [w1157 w1166] -> w1140
              tunnel: w1117 -> [w1157 w1166]
              tunnel: w1139 -> [w1155 w1161]
              tunnel: w1138 -> [w1156 w1164]
              tunnel: [w1156 w1165] -> w1137
              tunnel: [w1155 w1162] -> w1136
              tunnel: w1113 -> [_ w1163]
              tunnel: [w1154 w1158] -> w1127
              frame False {
              }
              frame True {
                # "new section in table\n--> add header row"
                n482 = Build Array("") -> (w1159:string[])
                n483 = Build Array (concatenate)(w1164, w1163) -> (w1165:string[])
                n484 = Build Array (concatenate)(w1161, w1159) -> (w1162:string[][])
              }
            }
            n485 = Format Into String(format string=w1114, w1121) -> (resulting string=w1129:string)  [unwired: 2 in, 1 out]
            n486 = call-poly <vilib>:"SVFA Get Spectrum Value.vi"("spectra"=w1123, "x value (1000)"=w1121, "coercion (nearest)"=w1148, "spectrum info"=w1122) -> ("spectra values"=w1147:dbl[], "actual x values"=w1124:dbl[])  [unwired: 11 in, 3 out]
            n487 = case shown="\"Band\", \"Differential\", \"Integral\", \"Pair\"" w1113 {
              selector: w1113 -> [w1174 _ _]
              tunnel: w1147 -> [w1176 w1213 w1251]
              tunnel: w1137 -> [w1182 w1217 w1256]
              tunnel: w1140 -> [w1181 w1216 w1250]
              tunnel: [w1180 w1215 w1249] -> w1146
              tunnel: w1136 -> [w1170 w1200 w1255]
              tunnel: [w1179 w1214 w1246] -> w1145
              tunnel: w1130 -> [_ w1212 _]
              tunnel: w1129 -> [w1173 w1207 w1253]
              tunnel: w1128 -> [w1177 w1202 w1241]
              tunnel: w1127 -> [w1168 w1201 _]
              tunnel: w1126 -> [_ w1197 _]
              tunnel: w1114 -> [w1172 _ _]
              tunnel: w1125 -> [w1171 _ _]
              tunnel: w1124 -> [_ _ w1245]
              tunnel: w1123 -> [_ _ w1240]
              tunnel: w1122 -> [_ _ w1239]
              frame Default {
                n488 = case shown="\"Sideband\"" w1174 {
                  tunnel: w1172 -> [_ w1192]
                  tunnel: w1171 -> [_ w1191]
                  tunnel: [_ w1190] -> w1167
                  frame Default {
                  }
                  frame "Sideband" {
                    n489 = Format Value(string ("")="s=", format string=w1192, value (0)=w1191) -> (output string=w1190:string)
                  }
                }
                n490 = case shown="True" w1168 {
                  tunnel: w1170 -> [w1183 w1187]
                  tunnel: [w1183 w1189] -> w1169
                  tunnel: w1167 -> [_ w1185]
                  frame False {
                  }
                  frame True {
                    n491 = Matrix Size(0:w1187) -> (1:w1188:i32)  [unwired: 1 out]
                    n492 = Decrement(x=w1188) -> (x-1=w1186:i32)
                    n493 = Replace Array Subset(array=w1187, new element=w1185, index (row)=w1186, index (col)=0 ("disabled index (col)")) -> (w1189:string[][])
                  }
                }
                n494 = for {
                  tunnel: w1176 -> [w1196] mode=indexing
                  tunnel: [w1195] -> w1178 mode=indexing
                  tunnel: w1177 -> [w1194]
                  n495 = Format Value(format string=w1194, value (0)=w1196) -> (output string=w1195:string)  [unwired: 1 in]
                }
                n496 = Build Array (concatenate)(w1173, w1178) -> (w1175:string[])
                n497 = Build Array (concatenate)(w1182, w1181) -> (w1180:string[])
                n498 = Build Array (concatenate)(w1169, w1175) -> (w1179:string[][])
              }
              frame "XY" {
                n499 = Get Variant Attribute(Variant=w1212, name="xy type", default value (empty Variant)=u16 0 ("precision (6)")) -> (duplicate Variant=w1211:variant, value=w1208:u16)  [unwired: 1 in, 2 out]
                n500 = case shown="1" w1208 {
                  tunnel: [0.0 ("element") w1233] -> w1205
                  tunnel: w1211 -> [_ w1236]
                  tunnel: w1202 -> [_ w1234]
                  tunnel: [_ w1232] -> w1198
                  frame 0, Default {
                  }
                  frame 1 {
                    n501 = Get Variant Attribute(Variant=w1236, name="y reference", default value (empty Variant)=0.0 ("element")) -> (value=w1233:dbl)  [unwired: 1 in, 3 out]
                    n502 = Format Value(string ("")="ref=", format string=w1234, value (0)=w1233) -> (output string=w1232:string)
                  }
                }
                n503 = case shown="True" w1201 {
                  tunnel: w1200 -> [w1218 w1223]
                  tunnel: [w1218 w1227] -> w1199
                  tunnel: w1198 -> [_ w1226]
                  tunnel: w1197 -> [_ w1225]
                  frame False {
                  }
                  frame True {
                    n504 = Initialize Array(w1226, w1225) -> (w1221:string[])
                    n505 = Matrix Size(0:w1223) -> (1:w1224:i32)  [unwired: 1 out]
                    n506 = Build Array (concatenate)("", w1221) -> (w1219:string[])
                    n507 = Decrement(x=w1224) -> (x-1=w1222:i32)
                    n508 = Replace Array Subset(array=w1223, new element=w1219, index (row)=w1222) -> (w1227:string[][])  [unwired: 1 in]
                  }
                }
                n509 = Subtract(x=w1213, y=w1205) -> (x-y=w1204:dbl[])
                n510 = for {
                  tunnel: w1204 -> [w1230] mode=indexing
                  tunnel: [w1229] -> w1203 mode=indexing
                  tunnel: w1202 -> [w1228]
                  n511 = Format Value(format string=w1228, value (0)=w1230) -> (output string=w1229:string)  [unwired: 1 in]
                }
                n512 = Build Array (concatenate)(w1207, w1203) -> (w1206:string[])
                n513 = Build Array (concatenate)(w1217, w1216) -> (w1215:string[])
                n514 = Build Array (concatenate)(w1199, w1206) -> (w1214:string[][])
              }
              frame "Band", "Differential", "Integral", "Pair" {
                n515 = for {
                  tunnel: w1251 -> [w1311] mode=indexing
                  tunnel: [w1310] -> w1254 mode=indexing
                  tunnel: w1241 -> [w1309]
                  n516 = Format Value(format string=w1309, value (0)=w1311) -> (output string=w1310:string)  [unwired: 1 in]
                }
                n517 = Index Array(array=w1245) -> (element=w1244:dbl)  [unwired: 1 in]
                n518 = Build Array (concatenate)(w1253, w1254) -> (w1252:string[])
                n519 = Build Array (concatenate)(w1244, w1251) -> (w1243:dbl[])
                n520 = Build Array (concatenate)(w1256, w1250) -> (w1248:string[])
                n521 = Build Array (concatenate)(w1255, w1252) -> (w1247:string[][])
                n522 = feedback-in #12(w1243) -> ()
                n523 = feedback #12() -> (w1242:dbl[])  [unwired: 1 in]
                n524 = case shown="\"B2\"" w1250 {
                  tunnel: [w1258 w1308] -> w1249
                  tunnel: w1248 -> [w1280 w1308]
                  tunnel: w1247 -> [w1278 w1307]
                  tunnel: [w1257 w1307] -> w1246
                  tunnel: w1243 -> [w1265 _]
                  tunnel: w1242 -> [w1267 _]
                  tunnel: w1241 -> [w1276 _]
                  tunnel: w1240 -> [w1270 _]
                  tunnel: w1239 -> [w1269 _]
                  frame "B2" {
                    n525 = Subtract(x=w1265, y=w1267) -> (x-y=w1274:dbl[])
                    n526 = Index Array(array=w1267) -> (element=w1266:dbl)  [unwired: 1 in]
                    n527 = Index Array(array=w1265) -> (element=w1264:dbl)  [unwired: 1 in]
                    n528 = Index Array(array=w1274) -> (element=w1275:dbl)  [unwired: 1 in]
                    n529 = Bundle By Name(cluster=cluster{"start":dbl, "stop":dbl} {"start"=-1.0, "stop"=-1.0} ("range"), "start"=w1266, "stop"=w1264) -> (w1268:cluster{"start":dbl, "stop":dbl})
                    n530 = Divide(x=w1274, y=w1275) -> (x/y=w1273:dbl[])
                    n531 = call-poly <vilib>:"SVFA Get Spectrum Subset.vi"("spectra"=w1270, "range"=w1268, "spectrum info"=w1269) -> ("spectra subsets"=w1263:cluster{"x0":dbl, "dx":dbl, "magnitude":dbl[]}[], "actual ranges"=w1260:cluster{"start":dbl, "stop":dbl}[])  [unwired: 11 in, 4 out]
                    n532 = for {
                      tunnel: w1274 -> [w1289] mode=indexing
                      tunnel: [w1288] -> w1277 mode=indexing
                      tunnel: w1276 -> [w1283]
                      tunnel: w1273 -> [w1287] mode=indexing
                      tunnel: [w1286] -> w1272 mode=indexing
                      tunnel: w1263 -> [w1284]
                      tunnel: [w1282] -> w1262 mode=indexing
                      tunnel: w1260 -> [w1281]
                      i -> [w1285]
                      n533 = case shown="Default" w1285 {
                        selector: w1285 -> [_ w1306]
                        tunnel: w1284 -> [_ w1305]
                        tunnel: w1283 -> [w1292 w1304]
                        tunnel: [w1291 w1303] -> w1282
                        tunnel: w1281 -> [w1298 _]
                        frame 0 {
                          n534 = Index Array(array=w1298) -> (element=w1290:cluster{"start":dbl, "stop":dbl})  [unwired: 1 in]
                          n535 = Unbundle(w1290) -> ("start"=w1297:dbl, "stop"=w1296:dbl)
                          n536 = Compound Arithmetic op=ADD(w1297, w1296) -> (w1295:dbl)
                          n537 = Compound Arithmetic op=MULTIPLY(w1295, 0.5 ("value")) -> (w1293:dbl)
                          n538 = Format Value(format string=w1292, value (0)=w1293) -> (output string=w1291:string)  [unwired: 1 in]
                        }
                        frame Default {
                          n539 = Decrement(x=w1306) -> (x-1=w1299:i32)
                          n540 = Index Array(array=w1305, index=w1299) -> (element=w1302:cluster{"x0":dbl, "dx":dbl, "magnitude":dbl[]})
                          n541 = Unbundle(w1302) -> ("magnitude"=w1301:dbl[])  [unwired: 2 out]
                          n542 = call-poly <vilib>:"Mean.vi"("X"=w1301) -> ("mean"=w1300:dbl)  [unwired: 1 out]
                          n543 = Format Value(format string=w1304, value (0)=w1300) -> (output string=w1303:string)  [unwired: 1 in]
                        }
                      }
                      n544 = Format Value(format string=w1283, value (0)=w1289) -> (output string=w1288:string)  [unwired: 1 in]
                      n545 = Format Value(format string=w1283, value (0)=w1287) -> (output string=w1286:string)  [unwired: 1 in]
                    }
                    n546 = Build Array (concatenate)(w1280, "b2-b1", "dy/dx", "average in band") -> (w1258:string[])
                    n547 = Build Array (concatenate)(w1278, w1277, w1272, w1262) -> (w1257:string[][])
                  }
                  frame "B1", Default {
                  }
                }
              }
            }
          }
        }
      }
    }
  }
  "channels" <- w5
  "measurement names" <- w3
  "value table" <- w4
  "Display State Out" <- w10
  n548 = property class="Tbl"(reference=w6, "Column Headers[]"=w5, "Row Headers[]"=w3, "Value"=w4) -> ()  [unwired: 1 in, 2 out]
